vi "Periodic Tasks.vi"(8 "error in":errorcluster) -> ()   [LabVIEW 2015]
doc: "This VI runs in parallel to other tasks. It can contain as many user-defined periodic loops as you need. These can carry out PID or other sorts of timed response."
uses:
  PID Constants.ctl
  Pneumatic State Machine.ctl
  DriveStates.ctl
  DriveTypes.ctl
  Auto Control.ctl
  <vilib>/Rock Robotics/WPI/DriverStation/WPI_DriverStationAllianceInfo.ctl
  <vilib>/Rock Robotics/WPI/DriverStation/WPI_DriverStationPositionInfo.ctl
  IMUType.ctl
  <vilib>/Platform/TimedLoop/XDataNode/timing_clust.ctl
  <vilib>/Platform/TimedLoop/XDataNode/nitl_modes.ctl
  <vilib>/Platform/TimedLoop/XDataNode/wakeup.ctl
  <vilib>/Rock Robotics/WPI/Solenoid/WPI_SolenoidValue.ctl
  Pneumatic Commands.ctl
  <vilib>/Rock Robotics/WPI/DriverStation/WPI_DriverStationRobotMode2.ctl
  <vilib>/Rock Robotics/WPI/Utilities/WPI_GetSetVariantRefNum.vi
  <vilib>/Rock Robotics/WPI/Solenoid/WPI_SolenoidSetEnum.vi
  <vilib>/Rock Robotics/Network Tables/NT Write Boolean.vi
  <vilib>/Rock Robotics/Network Tables/NT Write Number.vi
  <vilib>/platform/TimedLoop/XDataNode/XDataNode.xnode
  <vilib>/addons/control/pid/NI_PID_pid.lvlib
  <vilib>/Platform/TimedLoop/XDataNode/XDNodeRunTimeDep.lvlib
  <vilib>/addons/control/pid/pid.llb/PID Output Rate Limiter (DBL).vi
  <vilib>/Rock Robotics/Network Tables/NT Read String.vi
panel:
  out "IMU Type":T1
  out "Analog Pitch Gyro 2":dbl(graph)=-229.6875
  in  "Alt imu":bool
  in  "PImu fail":bool
  out "Climb State":T2=enum."Up and Float"
  in  "Reload QCP":bool
  out "Position":T3
  out "Alliance":T4
  out "Distance Remaining 2":dbl
  out "Motor Current":dbl(graph)=12.625
  in  "Tab Control":T5(tab)=enum."Drive"
  out "Waveform Chart":cluster{"Double":dbl, "Double":dbl}(graph)
  in  "cluster 2":T6={"Command"=enum."Stop", "Distance"=70.0, "Angle"=75.0, "Power"=0.6}
  in  "Send Command 2":bool
  out "Auto Command":T7
  in  "Tollerances":T8={"Evaluation Period"=0.5, "Dead Zone"=1.0, "Throttle Scale"=0.7}
  in  "Drive Mode":u32
  in  "real mode":bool=TRUE
  out "Distance Remaining":dbl=100.0
  out "Delta Angle Remaining 2":dbl=0.3125
  out "Distance":T9(graph)
  out "Angle":cluster{"Angle Setpoint":dbl, "Yaw":dbl}(graph)={"Angle Setpoint"=87.11416811253483, "Yaw"=3.4375}
  in  "Negates":T10={"negate turn"=TRUE, "negate throttle"=FALSE}
  in  "Throttle Scale":dbl(knob)=0.6332538458134985 scale=0.0..1.0
  in  "Distance Delta":dbl=10.0
  in  "Angle Delta":dbl(knob)=83.67666811253483 scale=-100.0..100.0
  in  "output rate (EGU/min)":dbl(knob)=125.7747299198201 scale=0.0..200.0
  in  "Angle Wrap":bool
  in  "Eval Period (sec)":dbl(knob)=0.503724380465646 scale=0.0..1.0
  in  "tol":dbl=0.5 format="%#_13g"
  out "Shoot":bool
  in  "Period":i64=20
  out "Late?":bool
  out "Delta Angle Remaining":dbl=83.67666811253483
  in  "output range":cluster{"output high":dbl, "output low":dbl}={"output high"=1.0, "output low"=-1.0}
  out "Delta Angle Remaining 3":dbl
  out "Drive Mode 2":T11
  in  "PID Constants":T12={"Drive Distance PID"={"proportional gain (Kc)"=0.2, "integral time (Ti, min)"=0.0, "derivative time (Td, min)"=0.001}, "Drive Straight PID"={"proportional gain (Kc)"=0.035, "integral time (Ti, min)"=0.0, "derivative time (Td, min)"=0.0008}, "TurnPID"={"proportional gain (Kc)"=0.07, "integral time (Ti, min)"=0.005, "derivative time (Td, min)"=0.0008}, "Hold Position PID"={"proportional gain (Kc)"=0.2, "integral time (Ti, min)"=0.02, "derivative time (Td, min)"=0.001}} {"Hold Position PID"."derivative time (Td, min)" format="%.10f"; "Hold Position PID"."integral time (Ti, min)" format="%.8f"; "Hold Position PID"."proportional gain (Kc)" format="%.3f"; "TurnPID"."derivative time (Td, min)" format="%.6f"; "TurnPID"."integral time (Ti, min)" format="%.10f"; "TurnPID"."proportional gain (Kc)" format="%.6f"; "Drive Straight PID"."derivative time (Td, min)" format="%.6f"; "Drive Straight PID"."integral time (Ti, min)" format="%.10f"; "Drive Straight PID"."proportional gain (Kc)" format="%.6f"; "Drive Distance PID"."derivative time (Td, min)" format="%.10f"; "Drive Distance PID"."integral time (Ti, min)" format="%.8f"; "Drive Distance PID"."proportional gain (Kc)" format="%.3f"}
  out "M":T13={"Boolean"=FALSE, "Boolean 2"=FALSE, "Boolean 3"=FALSE, "Boolean 4"=TRUE}
  out "A":T13={"Boolean"=FALSE, "Boolean 2"=FALSE, "Boolean 3"=TRUE, "Boolean 4"=FALSE}
  out "G":T13={"Boolean"=TRUE, "Boolean 2"=FALSE, "Boolean 3"=FALSE, "Boolean 4"=FALSE}
  out "S":T13={"Boolean"=FALSE, "Boolean 2"=FALSE, "Boolean 3"=FALSE, "Boolean 4"=TRUE}
  out "Analog Yaw Gyro":dbl(graph)=-229.6875
  in  "Read Enable":T14={"Cal Status"=TRUE, "Orientation"=TRUE, "Gyro"=FALSE, "Accelerometer"=FALSE, "Quanterion"=FALSE, "Accel Mode"=enum."Linear", "Magnetometer"=FALSE}
  out "Yaw":dbl(graph)=37.4375
  out "Pitch":dbl(graph)=1.75
  out "Roll":dbl(graph)=0.5
  out "X Acc":dbl
  out "Y Acc":dbl
  out "Z Acc":dbl
  out "Anomaly":bool
  in  "Earth Field (uT)":cluster{"Earth":dbl, "Tolerance":dbl}={"Earth"=51.0, "Tolerance"=5.0}
  out "Mag Vector":dbl
  out "IMUStatus":bool
  out "Late? 2":bool
  in  "Sensor Period":i64=20
  out "pitch":dbl=1.75
  in  "Max Val":dbl(knob)=1.0 scale=0.5..1.0
  in  "Offset 2":dbl(knob)=0.6008653928286186 scale=0.0..1.0
  in  "Dead Zone 2":dbl(knob)=0.09984207295572244 scale=0.0..1.0
  in  "Offset":dbl(knob)=0.267936230826254 scale=0.0..1.0
  in  "Dead Zone":dbl(knob)=0.10126960022109426 scale=0.0..1.0
  out "Left Encoder Distance":dbl=4402.950615
  out "Right Encoder Distance":dbl
  in  "Reset Encoders":bool
  out "Intake Chart":dbl(graph)=3.0
  out "Intake State":T2=enum."Up and Float"
  out "Tusk State":T2=enum."Up and Float"
  in  "a parameter too":dbl=0.5 format="%#_13g"
  in  "dist away":dbl=20.0 format="%#_13g"
  out "pitch 2":dbl=1.75
  out "Mag Vector 2":dbl
  out "Anomaly 2":bool
  in  "Earth Field (uT) 2":cluster{"Earth":dbl, "Tolerance":dbl}={"Earth"=51.0, "Tolerance"=5.0}
  out "Z Acc 2":dbl
  out "Y Acc 2":dbl
  out "X Acc 2":dbl
  out "M 2":T13={"Boolean"=FALSE, "Boolean 2"=FALSE, "Boolean 3"=FALSE, "Boolean 4"=TRUE}
  out "A 2":T13={"Boolean"=FALSE, "Boolean 2"=FALSE, "Boolean 3"=TRUE, "Boolean 4"=FALSE}
  out "G 2":T13={"Boolean"=TRUE, "Boolean 2"=FALSE, "Boolean 3"=FALSE, "Boolean 4"=FALSE}
  out "S 2":T13={"Boolean"=FALSE, "Boolean 2"=FALSE, "Boolean 3"=FALSE, "Boolean 4"=TRUE}
  in  "Read Enable 2":T14={"Cal Status"=TRUE, "Orientation"=TRUE, "Gyro"=FALSE, "Accelerometer"=FALSE, "Quanterion"=FALSE, "Accel Mode"=enum."Linear", "Magnetometer"=FALSE}
  # "Bazemore\nStraight Gains\nP=0.035\nI=0.00\nD=0.0008"
  # "Cass\nHold Position\nGains\nP=0.2\nI=0.02\nD=0.001"
  # "Bazemore\nTurn Gains\nP=0.07\nI=0.005\nD=0.0008"
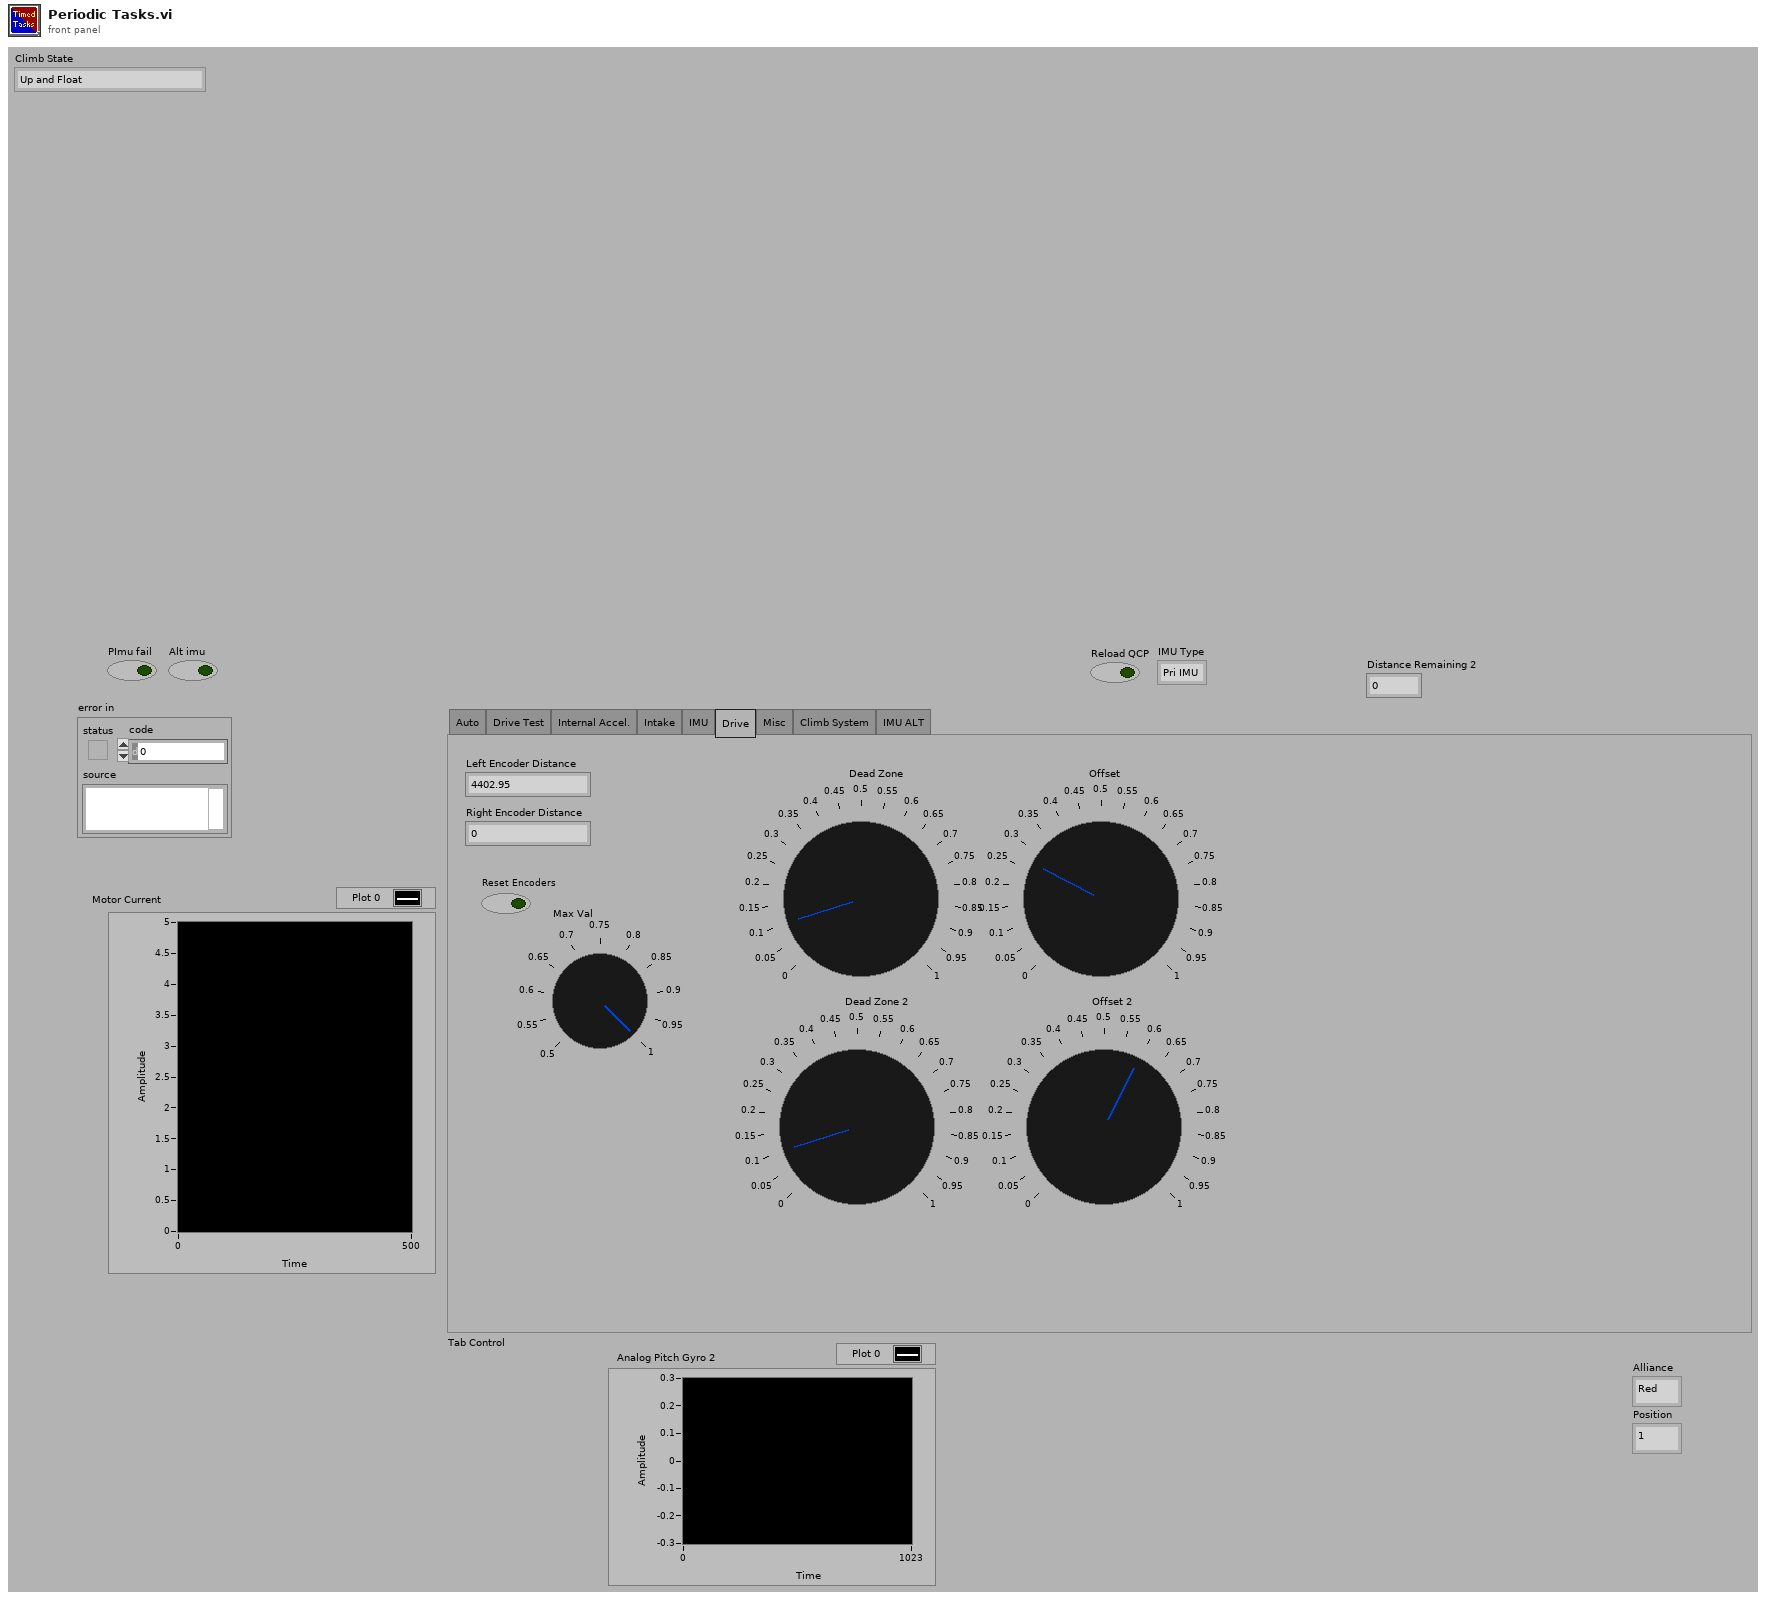
[diagram p1: front panel]
types:
  T1 = typedef "IMUType.ctl" = enum16{"Pri IMU", "Alt IMU", "Analog GYRO"}
  T2 = typedef "Pneumatic State Machine.ctl" = enum16{"Up and Pressure", "Down and Pressue", "Up and Float", "Down and Float"}
  T3 = typedef "WPI_DriverStationPositionInfo.ctl" = enum16{"1", "2", "3"}
  T4 = typedef "WPI_DriverStationAllianceInfo.ctl" = enum16{"Red", "Blue", "Invalid"}
  T5 = enum32{"Auto", "Drive Test", "Internal Accel.", "Intake", "IMU", "Drive", "Misc", "Climb System", "IMU ALT"}
  T6 = typedef "Auto Control.ctl" = cluster{"Command":T7, "Distance":dbl, "Angle":dbl, "Power":dbl}
  T7 = typedef "DriveStates.ctl" = enum16{"Wait for Notification", "Drive for Distance", "Drive Continuous", "Drive Absolute Heading", "Drive Relative Heading", "Turn Continuous", "Turn Degree", "Stop", "Follow Camera", "Hold Position"}
  T8 = cluster{"Evaluation Period":dbl, "Dead Zone":dbl, "Throttle Scale":dbl}
  T9 = cluster{"Distance Setpoint":dbl, "Desired Distance":dbl}
  T10 = cluster{"negate turn":bool, "negate throttle":bool}
  T11 = typedef "DriveTypes.ctl" = enum16{"Auto Turn", "Auto Straight", "Auto Vision Align"}
  T12 = typedef "PID Constants.ctl" = cluster{"Drive Distance PID":cluster{"proportional gain (Kc)":dbl, "integral time (Ti, min)":dbl, "derivative time (Td, min)":dbl}, "Drive Straight PID":cluster{"proportional gain (Kc)":dbl, "integral time (Ti, min)":dbl, "derivative time (Td, min)":dbl}, "TurnPID":cluster{"proportional gain (Kc)":dbl, "integral time (Ti, min)":dbl, "derivative time (Td, min)":dbl}, "Hold Position PID":cluster{"proportional gain (Kc)":dbl, "integral time (Ti, min)":dbl, "derivative time (Td, min)":dbl}}
  T13 = cluster{"Boolean":bool, "Boolean 2":bool, "Boolean 3":bool, "Boolean 4":bool}
  T14 = cluster{"Cal Status":bool, "Orientation":bool, "Gyro":bool, "Accelerometer":bool, "Quanterion":bool, "Accel Mode":enum8{"Raw Data", "Linear", "Gravity"}, "Magnetometer":bool}
  T15 = cluster{"Yaw Wind":dbl, "Roll Wind":dbl, "Pitch Wind":dbl}
  T16 = typedef "WPI_DriverStationRobotMode2.ctl" = enum16{"Autonomous Disabled", "Autonomous Enabled", "Teleop Disabled", "Teleop Enabled", "Disconnected", "Finish", "Test Disabled", "Test Enabled", "Emergency Stopped"}
  T17 = typedef "Pneumatic Commands.ctl" = enum16{"Go Up", "Go Down", "Nothing"}
  T18 = typedef "WPI_SolenoidValue.ctl" = enum16{"Off", "On", "Forward", "Reverse"}
  T19 = cluster{"tdms":refnum<k34>, "Channel IDs":string[], "TDMS Name":string, "Burst Size":i32, "Que":refnum<k33>, "Default Array":dbl[], "occurrence":refnum<k4>}
  T20 = typedef "XDNodeRunTimeDep.lvlib/timing_clust.ctl" = cluster{"Expected End [f-1]":u64, "Actual End [f-1]":u64, "Finished Late? [f-1]":bool, "Expected End [i-1]":u64, "Actual End [i-1]":u64, "Finished Late? [i-1]":bool, "Expected Start [i]":u64, "Actual Start [i]":u64, "Expected Start [f]":u64, "Actual Start [f]":u64, "Source Name":string, "Structure Name":string, "Period":i64, "Deadline":i64, "Offset":i64, "Start":i64, "Priority":i32, "Timeout":i32, "Mode":T21, "Wakeup Reason":T22, "Error":errorcluster, "Source Type":string, "Secondary Source Type":string, "Global End Time":u64, "Global Start Time":u64, "Frame Duration":u64, "Iteration Duration":u64, "Assigned CPU":i32, "I/O Scan Engine Mode":u32}
  T21 = typedef "XDNodeRunTimeDep.lvlib/nitl_modes.ctl" = enum32{"No Change", "Process missed periods, maintain original phase", "Discard missed periods, maintain original phase", "Process missed periods, ignore original phase", "Discard missed periods, ignore original phase"}
  T22 = typedef "XDNodeRunTimeDep.lvlib/wakeup.ctl" = enum32{"Normal", "Aborted", "Asynchronous wakeup", "Timing source error", "Timed loop error", "Timeout"}
  T23 = enum16{"Low Bar", "Rough Terrain", "Moat", "Rock Wall", "Cheval de Frise", "Portcullis", "Sally Port", "Drawbridge", "Ramparts"}
  T24 = typedef "WPI_JoystickDevRef.ctl" = cluster{"Device":T25}
  T25 = typedef "WPI_JoystickDeviceEnum.ctl" = enum16{"USB 0", "USB 1", "USB 2", "USB 3", "USB 4", "USB 5"}
  T26 = typedef "WPI_RobotDriveDevRef.ctl" = cluster{"DevStatus":errorcluster, "Motors[]":T27[], "Square Inputs":bool, "Max Output":dbl}
  T27 = typedef "WPI_MotorControlDeviceRef.ctl" = cluster{"DeviceStatus":errorcluster, "Type":T28, "PWM":cluster{"PWM Channel":T29, "DeadBand":T30}, "CAN":cluster{"Device Number":u8, "Control Mode":T31, "Semaphore":T32, "Max Vout":dbl, "TalonSRX Control Mode":T33}, "Invert":bool}
  T28 = typedef "WPI_MotorControlType.ctl" = enum16{"PWM", "CAN", "CANTalonSRX"}
  T29 = typedef "FPGA_DIOPWMChannel.ctl" = enum8{"PWM 0", "PWM 1", "PWM 2", "PWM 3", "PWM 4", "PWM 5", "PWM 6", "PWM 7", "PWM 8", "PWM 9", "PWM MXP 0", "PWM MXP 1", "PWM MXP 2", "PWM MXP 3", "PWM MXP 4", "PWM MXP 5", "PWM MXP 6", "PWM MXP 7", "PWM MXP 8", "PWM MXP 9", "Invalid"}
  T30 = typedef "WPI_PWMDeadband.ctl" = cluster{"Name":string, "maxPositivePwm":i32, "minPositivePwm":i32, "centerPwm":i32, "maxNegativePwm":i32, "minNegativePwm":i32, "angularRange":u16}
  T31 = typedef "WPI_CANJaguar_ControlMode.ctl" = enum8{"Percent VBus", "Current", "Speed", "Position", "Voltage"}
  T32 = typedef "Semaphore RefNum" = refnum<k1>
  T33 = typedef "WPI_CANTalonSRX_APIControlMode.ctl" = enum8{"Percent VBus", "Speed", "Position", "Slave", "Unchanged / Invalid", "Voltage Compensation", "Current", "Motion Profile"}
  T34 = cluster{"Delta":dbl, "Throttle Scale":dbl, "Current Angle":dbl, "Current Distance":dbl}
  T35 = cluster{"Buttons[0]":bool, "Buttons[1]":bool, "Buttons[2]":bool, "Buttons[3]":bool, "Buttons[4]":bool, "Buttons[5]":bool, "Buttons[6]":bool, "Buttons[7]":bool, "Buttons[8]":bool}
  T36 = cluster{"Axes[0]":dbl, "Axes[1]":dbl, "Axes[2]":dbl, "Axes[3]":dbl, "Axes[4]":dbl, "Axes[5]":dbl, "Axes[6]":dbl, "Axes[7]":dbl, "Axes[8]":dbl}
  T37 = cluster{"proportional gain (Kc)":dbl, "integral time (Ti, min)":dbl, "derivative time (Td, min)":dbl}
  T38 = cluster{"Drive Distance PID":cluster{"proportional gain (Kc)":dbl, "integral time (Ti, min)":dbl, "derivative time (Td, min)":dbl}, "Drive Straight PID":cluster{"proportional gain (Kc)":dbl, "integral time (Ti, min)":dbl, "derivative time (Td, min)":dbl}}
  T39 = cluster{"Angle Setpoint":dbl, "Distance Setpoint":dbl}
  T40 = cluster{"Distance Setpoint":dbl, "Current Distance":dbl}
  T41 = typedef "WPI_I2CDevRef.ctl" = cluster{"DevStatus":errorcluster, "Device Address":u8, "Handle":i32, "I2C Bus":T42}
  T42 = typedef "i2c_bus.ctl" = enum16{"I2C On-Board", "I2C MXP", "Invalid"}
  T43 = typedef "WPI_GyroDevRef.ctl" = cluster{"DevStatus":errorcluster, "Analog Channel":T44, "Offset":dbl, "Gain (VoltsPerDegree/Second)":dbl, "Gyro Type":enum16{"Analog", "XRS450"}, "Handle":i32, "SPI Bus":T45, "Device Found":bool, "Sample Rate":dbl, "Calibrate On Open":bool}
  T44 = typedef "FPGA_AIChannel.ctl" = enum8{"AI 0", "AI 1", "AI 2", "AI 3", "AI MXP 0", "AI MXP 1", "AI MXP 2", "AI MXP 3", "Invalid"}
  T45 = typedef "spi_bus.ctl" = enum16{"SPI On-Board, CS0", "SPI On-Board, CS1", "SPI On-Board, CS2", "SPI On-Board, CS3", "SPI MXP", "Invalid"}
  T46 = typedef "WPI_ServoDeviceRef.ctl" = cluster{"DeviceStatus":errorcluster, "PWM Channel":T29, "DeadBand":T30}
  T47 = typedef "WPI_SolenoidDevRef.ctl" = cluster{"DevStatus":errorcluster, "Pneumatics Control Module":u8, "Forward Solenoid Channel":T48, "Reverse Solenoid Channel":T48}
  T48 = typedef "WPI_SolenoidChannel.ctl" = enum8{"Solenoid 0", "Solenoid 1", "Solenoid 2", "Solenoid 3", "Solenoid 4", "Solenoid 5", "Solenoid 6", "Solenoid 7", "Invalid"}
  T49 = cluster{"Mag":cluster{"[0]":bool, "[1]":bool, "[2]":bool, "[3]":bool}, "Acc":cluster{"[0]":bool, "[1]":bool, "[2]":bool, "[3]":bool}, "Gyro":cluster{"[0]":bool, "[1]":bool, "[2]":bool, "[3]":bool}, "Sys":cluster{"[0]":bool, "[1]":bool, "[2]":bool, "[3]":bool}, "Status":bool}
  T50 = cluster{"Yaw":dbl, "Roll":dbl, "Pitch":dbl, "Yaw Wind":dbl, "Roll Wind":dbl, "Pitch Wind":dbl}
  T51 = cluster{"X Mag":dbl, "Y Mag":dbl, "Z Mag":dbl, "Anomaly":bool}
  T52 = cluster{"[0]":bool, "[1]":bool, "[2]":bool, "[3]":bool}
  T53 = typedef "WPI_EncoderDevRef.ctl" = cluster{"DevStatus":errorcluster, "EncoderIndex":T54, "CounterIndex":T55, "DistancePerCount":dbl, "Decoding Type":T56}
  T54 = typedef "FPGA_EncoderIdx.ctl" = enum8{"Enc 0", "Enc 1", "Enc 2", "Enc 3", "Enc 4", "Enc 5", "Enc 6", "Enc 7", "Invalid"}
  T55 = typedef "FPGA_CounterCtrSystemIndex.ctl" = enum8{"Ctr 0", "Ctr 1", "Ctr 2", "Ctr 3", "Ctr 4", "Ctr 5", "Ctr 6", "Ctr 7", "Invalid"}
  T56 = typedef "WPI_EncoderType.ctl" = enum16{"1x", "2x", "4x"}
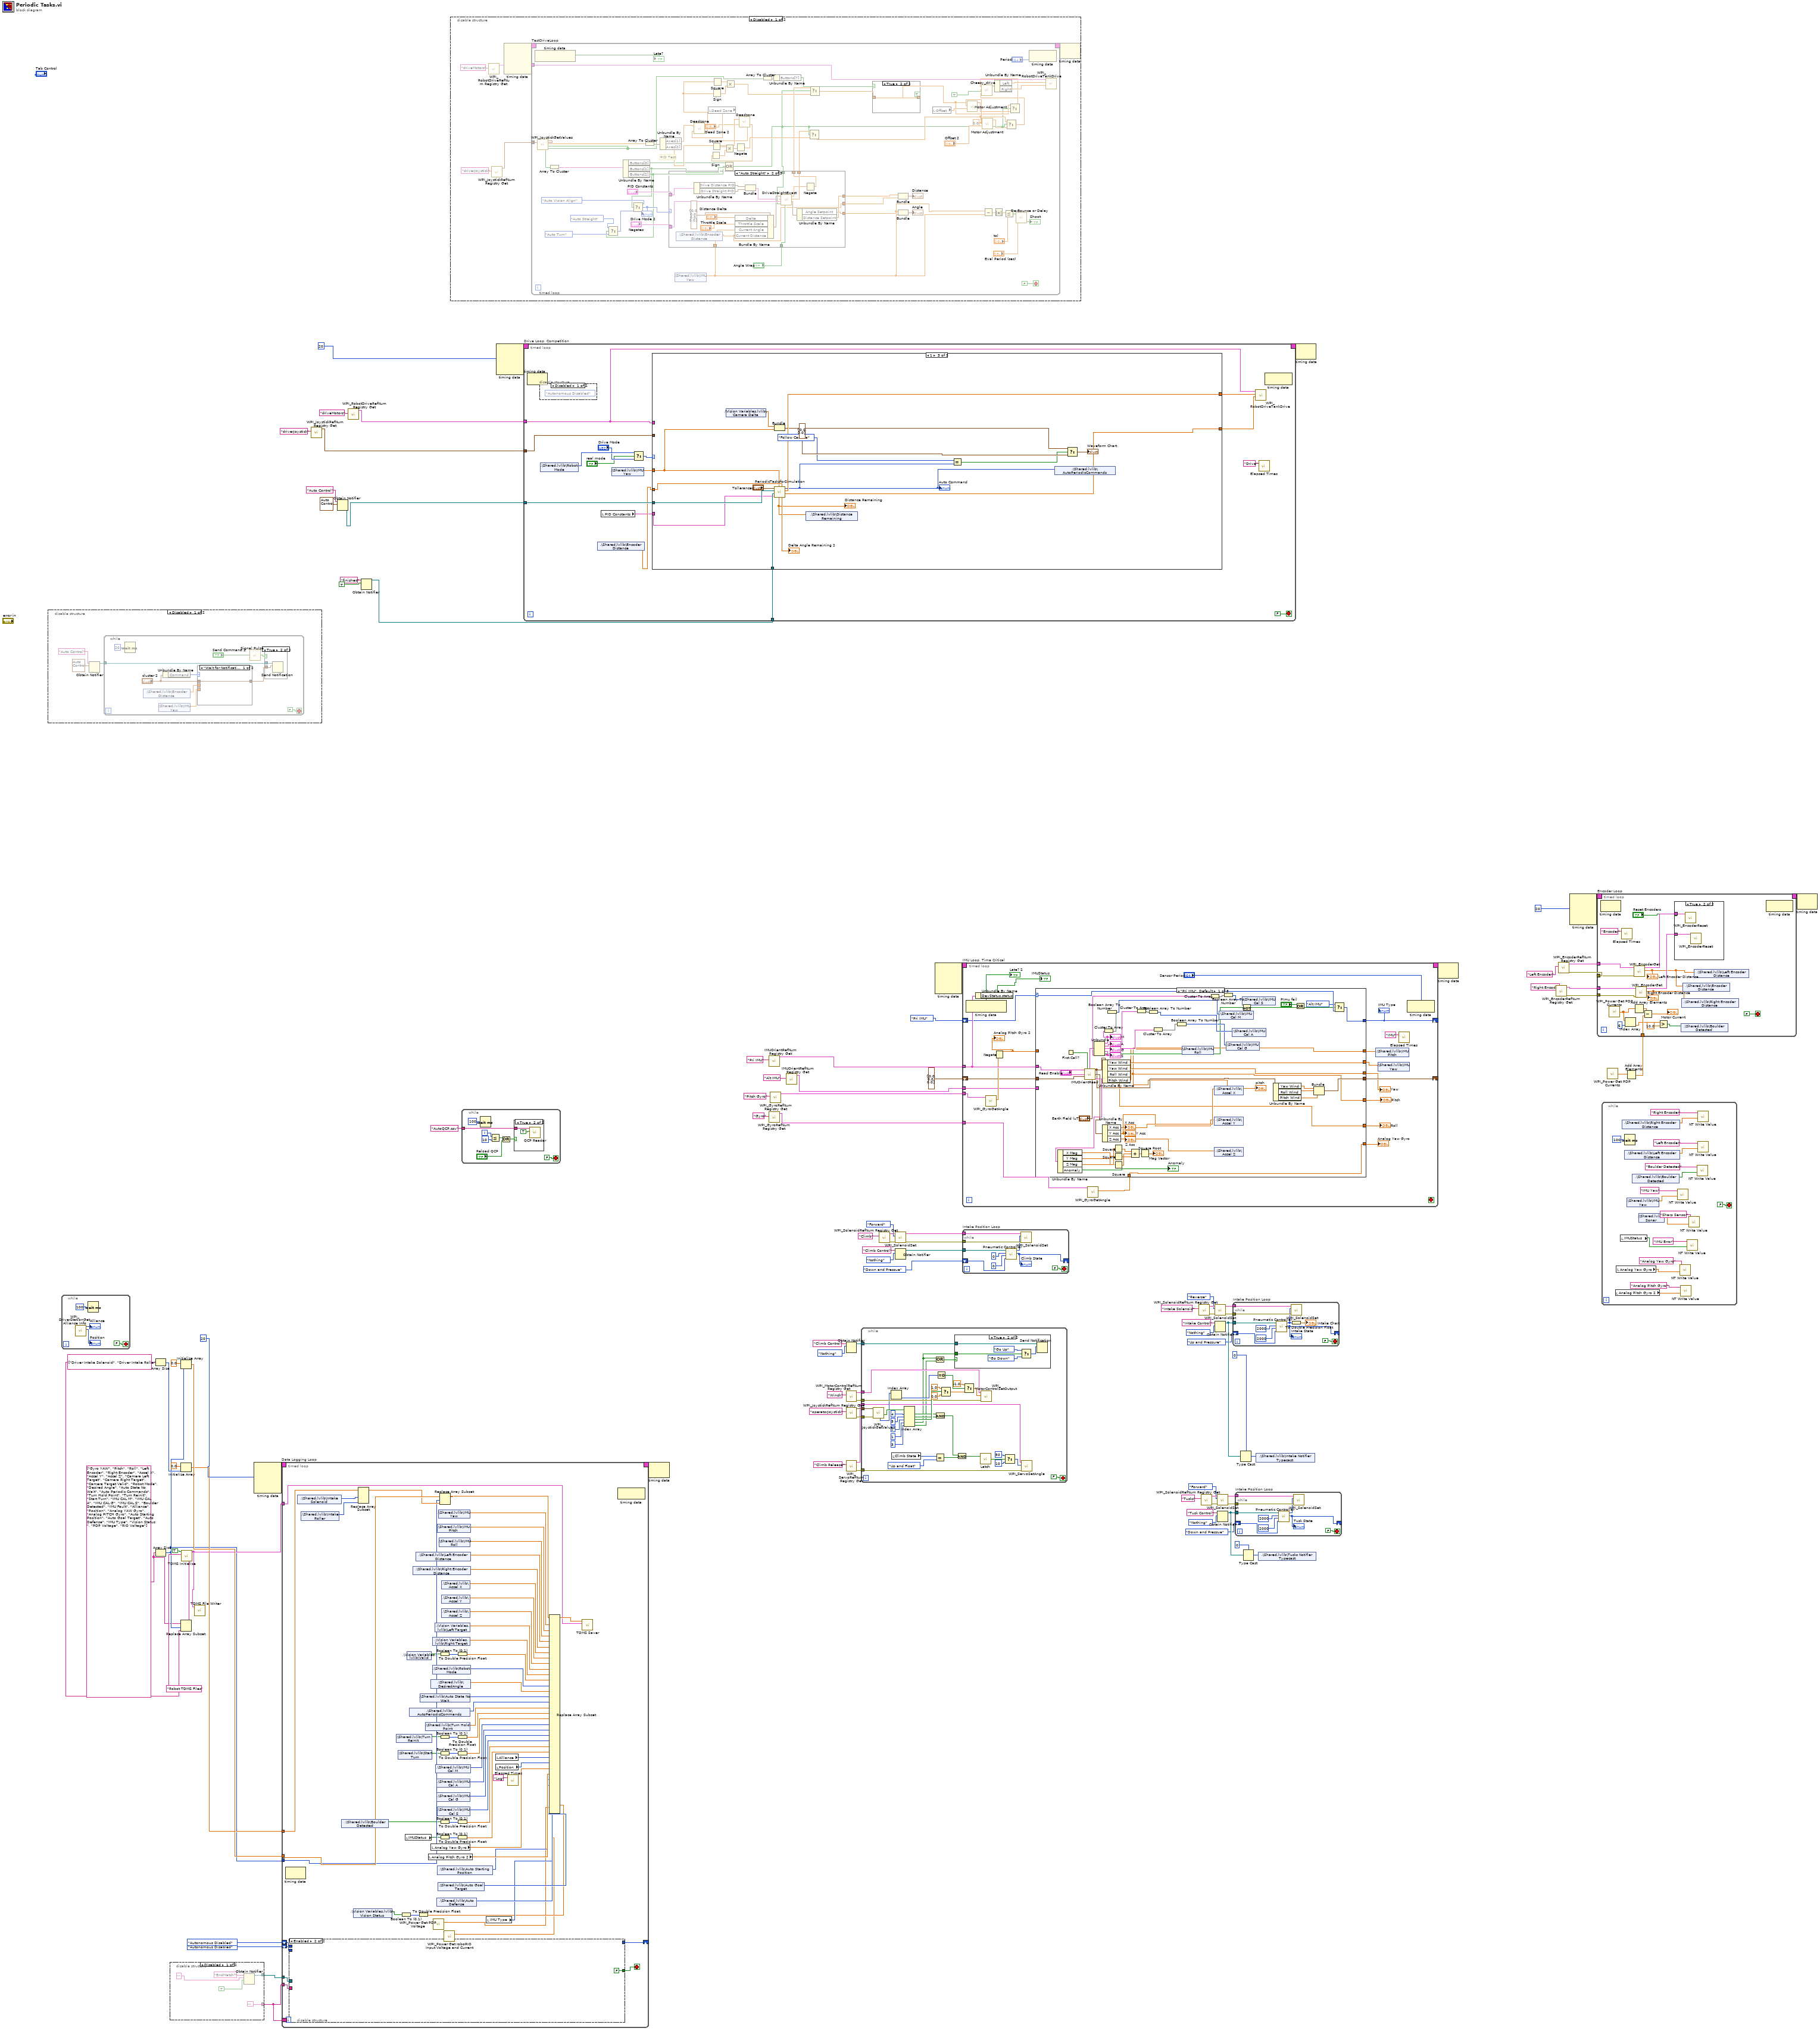
[diagram p0: block diagram]
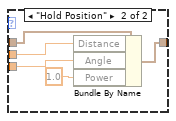
[diagram p4: hidden frame]
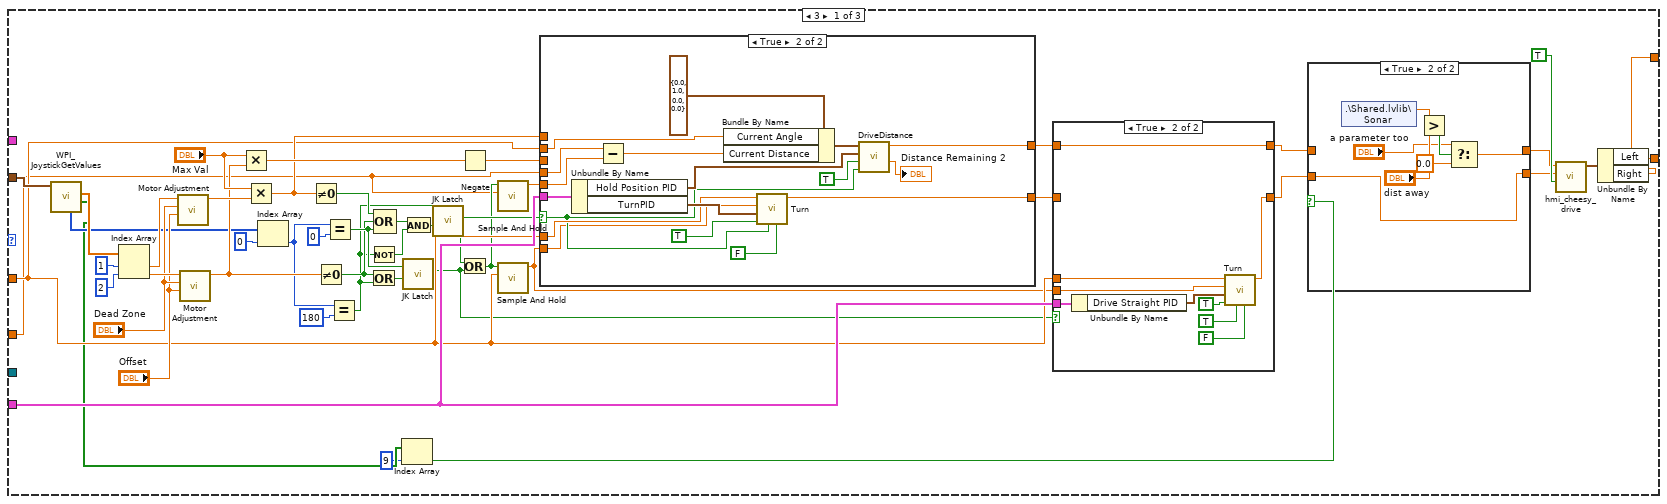
[diagram p9: hidden frame]
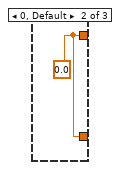
[diagram p13: hidden frame]
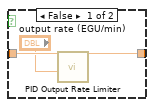
[diagram p14: hidden frame]
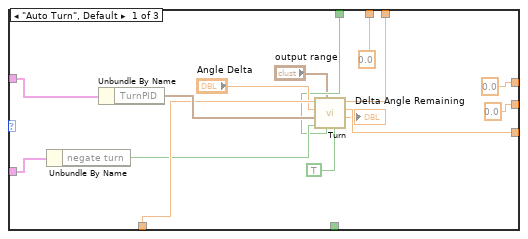
[diagram p15: hidden frame]
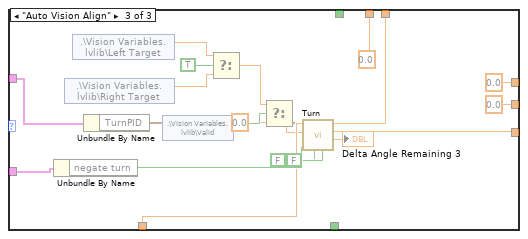
[diagram p16: hidden frame]
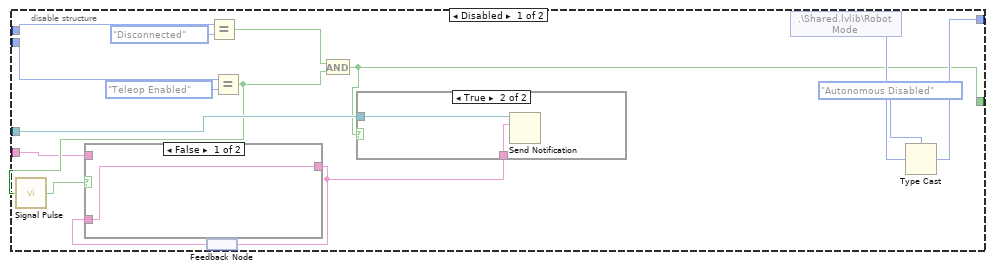
[diagram p19: hidden frame]
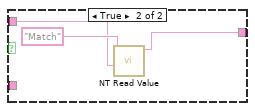
[diagram p20: hidden frame]
diagram:
  w1 = string[] ["Driver Intake Solenoid", "Driver Intake Roller"] ("Channel IDs")
  w3 = string[] ["Gyro YAW", "Pitch", "Roll", "Left Encoder", "Right Encoder", "Accel X", "Accel Y", "Accel Z", "Camera Left Target", "Camera Right Target", "Camera Target Valid", "Robot Mode", "Desired Angle", "Auto State No Wait", "Auto Periodic Commands", "Turn Hold Point", "Turn Reinit", "Start Turn", "IMU CAL M", "IMU CAL A", "IMU CAL G", "IMU CAL S", "Boulder Detected", "IMU Fault", "Alliance", "Position", "Analog YAW Gyro", "Analog PITCH Gyro", "Auto Starting Position", "Auto Goal Target", "Auto Defense", "IMU Type", "Vision Status ", "PDP Voltage", "RIO Voltage"] ("Channel IDs")
  n1 = disable-structure shown="Disabled" {
    frame Disabled {
      n2 = Obtain Notifier(name (unnamed)="Auto Control", notification data type=T6 {"Command"=enum."Drive for Distance", "Distance"=0.0, "Angle"=0.0, "Power"=0.0} ("cluster")) -> (notifier out=w103:refnum<notifier>)  [unwired: 2 in, 2 out]
      n3 = while {
        tunnel: w103 -> [w113]
        stop <- FALSE stop-if-true
        n4 = Wait (ms)(milliseconds to wait=u32 20) -> ()  [unwired: 1 out]
        n5 = shared-variable ".\\Shared.lvlib\\Encoder Distance"() -> (w107:dbl)  [unwired: 1 in, 1 out]
        n6 = shared-variable ".\\Shared.lvlib\\IMU Yaw"() -> (w106:dbl)  [unwired: 1 in, 1 out]
        n7 = Unbundle By Name("cluster 2") -> ("Command"=w110:T7)
        n8 = case shown="\"Wait for Notification\", Default" w110 {
          tunnel: "cluster 2" -> [w116 w121]
          tunnel: [w116 w120] -> w108
          tunnel: w107 -> [_ w119]
          tunnel: w106 -> [_ w118]
          frame "Wait for Notification", Default {
          }
          frame "Hold Position" {
            n9 = Bundle By Name(cluster=w121, "Distance"=w119, "Angle"=w118, "Power"=1.0) -> (w120:T6)
          }
        }
        n10 = call <userlib>:"Signal Pulse.vi"("Input"="Send Command 2") -> ("Output"=w114:bool)
        n11 = case shown="True" w114 {
          tunnel: w113 -> [_ w123]
          tunnel: w108 -> [_ w122]
          frame False {
          }
          frame True {
            n12 = Send Notification(notification=w122, notifier=w123) -> ()  [unwired: 1 in, 2 out]
          }
        }
      }
    }
    frame Enabled {
    }
  }
  n13 = while {
    stop <- FALSE stop-if-true
    n14 = call <vilib>:"WPI_DriverStationGet Alliance Info.vi"() -> ("Position"=→"Position":T3, "Alliance"=→"Alliance":T4)  [unwired: 10 in]
    n15 = Wait (ms)(milliseconds to wait=u32 100) -> ()  [unwired: 1 out]
  }
  n16 = Array Size(array=w1) -> (size(s)=w74:i32)
  n17 = Array Size(array=w3) -> (size(s)=w4:i32)
  n18 = disable-structure shown="Disabled" {
    disable-tunnel: [w130 _] -> w9
    disable-tunnel: ["" _] -> w8
    frame Disabled {
      n19 = Obtain Notifier(name (unnamed)="EndMatch?", notification data type="", create if not found? (T)=TRUE) -> (notifier out=w130:refnum<notifier>)  [unwired: 1 in, 2 out]
    }
    frame Enabled {
    }
  }
  n20 = Initialize Array(0.0, w4) -> (w89:dbl[])
  n21 = Initialize Array(0.0, w74) -> (w73:dbl[])
  n22 = Replace Array Subset(array=w3, new element=w1, index=w4) -> (w2:string[])
  n23 = call <userlib>:"TDMS Initialize.vi"("Channel IDs"=w2, "TDMS Name"="Robot TDMS Files", "Log to USB?"=TRUE) -> ("TDMS Cluster"=w5:T19)  [unwired: 8 in]
  n24 = call <userlib>:"TDMS File Writer.vi"("TDMS Cluster"=w5) -> ()  [unwired: 11 in]
  n25 = node-c288(i64 20 ("Period")) -> (w94:T20)  [unwired: 3 in]
  n26 = timed-loop "Data Logging Loop" {
    timing: w94 -> [_]
    timing-out: [_] -> w93
    tunnel: w5 -> [w170]
    tunnel: w89 -> [w186]
    tunnel: w73 -> [w184]
    tunnel: w4 -> [w182]
    shift-right: [w146] -> _
    shift-left: WPI_DriverStationRobotMode2."Autonomous Disabled" ("Robot Mode") -> [w148]
    shift-left: WPI_DriverStationRobotMode2."Autonomous Disabled" ("Robot Mode") -> [w147]
    tunnel: w9 -> [w145]
    border: w8 -> [_]
    tunnel: w8 -> [w143]
    stop <- w144 stop-if-true
    n27 = node-c288() -> ()  [unwired: 1 in, 1 out]
    n28 = disable-structure shown="Enabled" {
      disable-tunnel: w148 -> [w210 _]
      disable-tunnel: w147 -> [w209 _]
      disable-tunnel: [w207 _] -> w146
      disable-tunnel: w145 -> [w202 _]
      disable-tunnel: [w201 FALSE] -> w144
      disable-tunnel: w143 -> [w197 _]
      frame Disabled {
        n29 = feedback #1() -> (w198:string)
        n30 = Equal?(x=w210, y=WPI_DriverStationRobotMode2."Disconnected") -> (x = y?=w203:bool)
        n31 = Equal?(x=w209, y=WPI_DriverStationRobotMode2."Teleop Enabled") -> (x = y?=w200:bool)
        n32 = call <userlib>:"Signal Pulse.vi"("Input"=w200) -> ("Output"=w199:bool)
        n33 = case shown="False" w199 {
          tunnel: [w211 w213] -> w196
          tunnel: w197 -> [_ w212]
          tunnel: w198 -> [w211 _]
          frame False {
          }
          frame True {
            n34 = call-poly <vilib>:"NT Read Value.vi"("Default Value"=w212, "Name"="Match") -> ("String"=w213:string)  [unwired: 8 in, 1 out]
          }
        }
        n35 = feedback-in #1(w196) -> ()
        n36 = And(x=w203, y=w200) -> (x .and. y?=w201:bool)
        n37 = case shown="True" w201 {
          tunnel: w202 -> [_ w216]
          tunnel: w196 -> [_ w215]
          frame False {
          }
          frame True {
            n38 = Send Notification(notification=w215, notifier=w216) -> ()  [unwired: 1 in, 2 out]
          }
        }
        n39 = shared-variable ".\\Shared.lvlib\\Robot Mode"() -> (w208:u32)  [unwired: 1 in, 1 out]
        n40 = Type Cast(type=WPI_DriverStationRobotMode2."Autonomous Disabled" ("Robot Mode"), x=w208) -> (*(type *) &x=w207:T16)
      }
      frame Enabled {
      }
    }
    n41 = shared-variable ".\\Shared.lvlib\\Intake Solenoid"() -> (w181:u32)  [unwired: 1 in, 1 out]
    n42 = shared-variable ".\\Shared.lvlib\\Intake Roller"() -> (w180:u32)  [unwired: 1 in, 1 out]
    n43 = shared-variable ".\\Shared.lvlib\\Boulder Detected"() -> (w158:bool)  [unwired: 1 in, 1 out]
    n44 = shared-variable ".\\Vision Variables.lvlib\\Vision Status"() -> (w136:bool)  [unwired: 1 in, 1 out]
    n45 = Replace Array Subset(array=w184, new element #1=w181, new element #2=w180) -> (w183:dbl[])  [unwired: 2 in]
    n46 = shared-variable ".\\Shared.lvlib\\Turn Reinit"() -> (w167:bool)  [unwired: 1 in, 1 out]
    n47 = shared-variable ".\\Shared.lvlib\\Start Turn"() -> (w165:bool)  [unwired: 1 in, 1 out]
    n48 = Boolean To (0,1)(Boolean=w136) -> (0, 1=w137:i16)
    n49 = local read "IMUStatus"() -> (w151:bool)
    n50 = shared-variable ".\\Vision Variables.lvlib\\Valid"() -> (w177:bool)  [unwired: 1 in, 1 out]
    n51 = shared-variable ".\\Shared.lvlib\\AutoPeriodicCommands"() -> (w171:u16)  [unwired: 1 in, 1 out]
    n52 = shared-variable ".\\Shared.lvlib\\Right Encoder Distance"() -> (w190:dbl)  [unwired: 1 in, 1 out]
    n53 = shared-variable ".\\Shared.lvlib\\Left Encoder Distance"() -> (w191:dbl)  [unwired: 1 in, 1 out]
    n54 = To Double Precision Float(number=w137) -> (double precision float=w135:dbl)
    n55 = shared-variable ".\\Shared.lvlib\\Auto State No Wait"() -> (w172:u32)  [unwired: 1 in, 1 out]
    n56 = shared-variable ".\\Shared.lvlib\\Turn Hold Point"() -> (w169:dbl)  [unwired: 1 in, 1 out]
    n57 = local read "Analog Pitch Gyro 2"() -> (w142:dbl)
    n58 = shared-variable ".\\Shared.lvlib\\DesiredAngle"() -> (w173:dbl)  [unwired: 1 in, 1 out]
    n59 = local read "Analog Yaw Gyro"() -> (w149:dbl)
    n60 = shared-variable ".\\Vision Variables.lvlib\\Right Target"() -> (w178:dbl)  [unwired: 1 in, 1 out]
    n61 = shared-variable ".\\Shared.lvlib\\Robot Mode"() -> (w174:u32)  [unwired: 1 in, 1 out]
    n62 = call <vilib>:"WPI_Power Get PDP Voltage.vi"() -> ("voltage (V)"=w134:dbl)  [unwired: 14 in, 1 out]
    n63 = shared-variable ".\\Vision Variables.lvlib\\Left Target"() -> (w179:dbl)  [unwired: 1 in, 1 out]
    n64 = shared-variable ".\\Shared.lvlib\\IMU Cal M"() -> (w162:u32)  [unwired: 1 in, 1 out]
    n65 = shared-variable ".\\Shared.lvlib\\IMU Cal A"() -> (w161:u32)  [unwired: 1 in, 1 out]
    n66 = shared-variable ".\\Shared.lvlib\\IMU Cal G"() -> (w160:u32)  [unwired: 1 in, 1 out]
    n67 = shared-variable ".\\Shared.lvlib\\Auto Defense"() -> (w139:T23)  [unwired: 1 in, 1 out]
    n68 = shared-variable ".\\Shared.lvlib\\IMU Pitch"() -> (w193:dbl)  [unwired: 1 in, 1 out]
    n69 = shared-variable ".\\Shared.lvlib\\IMU Cal S"() -> (w159:u32)  [unwired: 1 in, 1 out]
    n70 = shared-variable ".\\Shared.lvlib\\Auto Starting Position"() -> (w141:enum16{"1", "2", "3", "4", "5"})  [unwired: 1 in, 1 out]
    n71 = shared-variable ".\\Shared.lvlib\\Auto Goal Target"() -> (w140:enum16{"Left Goal", "Right Goal", "Stop"})  [unwired: 1 in, 1 out]
    n72 = shared-variable ".\\Shared.lvlib\\IMU Yaw"() -> (w194:dbl)  [unwired: 1 in, 1 out]
    n73 = shared-variable ".\\Shared.lvlib\\IMU Roll"() -> (w192:dbl)  [unwired: 1 in, 1 out]
    n74 = Boolean To (0,1)(Boolean=w177) -> (0, 1=w176:i16)
    n75 = Boolean To (0,1)(Boolean=w167) -> (0, 1=w168:i16)
    n76 = Boolean To (0,1)(Boolean=w165) -> (0, 1=w166:i16)
    n77 = Boolean To (0,1)(Boolean=w158) -> (0, 1=w157:i16)
    n78 = Boolean To (0,1)(Boolean=w151) -> (0, 1=w152:i16)
    n79 = Replace Array Subset(array=w186, new element=w183, index=w182) -> (w185:dbl[])
    n80 = shared-variable ".\\Shared.lvlib\\Accel X"() -> (w189:dbl)  [unwired: 1 in, 1 out]
    n81 = shared-variable ".\\Shared.lvlib\\Accel Y"() -> (w188:dbl)  [unwired: 1 in, 1 out]
    n82 = shared-variable ".\\Shared.lvlib\\Accel Z"() -> (w187:dbl)  [unwired: 1 in, 1 out]
    n83 = call <vilib>:"WPI_Power Get roboRIO Input Voltage and Current.vi"() -> ("roboRIO input voltage (V)"=w133:dbl)  [unwired: 13 in, 2 out]
    n84 = To Double Precision Float(number=w176) -> (double precision float=w175:dbl)
    n85 = To Double Precision Float(number=w168) -> (double precision float=w164:dbl)
    n86 = To Double Precision Float(number=w166) -> (double precision float=w163:dbl)
    n87 = To Double Precision Float(number=w157) -> (double precision float=w156:dbl)
    n88 = To Double Precision Float(number=w152) -> (double precision float=w150:dbl)
    n89 = local read "IMU Type"() -> (w138:T1)
    n90 = local read "Alliance"() -> (w153:T4)
    n91 = local read "Position"() -> (w154:T3)
    n92 = call "Elapsed Times.vi"("Call Name"="Log") -> ()  [unwired: 2 in, 1 out]
    n93 = Replace Array Subset(array=w185, new element #1=w194, new element #2=w193, new element #3=w192, new element #4=w191, new element #5=w190, new element #6=w189, new element #7=w188, new element #8=w187, new element #9=w179, new element #10=w178, new element #11=w175, new element #12=w174, new element #13=w173, new element #14=w172, new element #15=w171, new element #16=w169, new element #17=w164, new element #18=w163, new element #19=w162, new element #20=w161, new element #21=w160, new element #22=w159, new element #23=w156, new element #24=w150, new element #25=w153, new element #26=w154, new element #27=w149, new element #28=w142, new element #29=w141, new element #30=w140, new element #31=w139, new element #32=w138, new element #33=w135, new element #34=w134, new element #35=w133) -> (w195:dbl[])  [unwired: 35 in]
    n94 = call <userlib>:"TDMS Saver.vi"("TDMS Cluster"=w170, "Data to Log"=w195) -> ()  [unwired: 10 in]
    n95 = node-c288() -> ()  [unwired: 1 in, 1 out]
  }
  n96 = call <vilib>:"WPI_JoystickRefNum Registry Get.vi"("refnum name"="driverJoystick") -> ("JoystickDevRef"=w62:T24)  [unwired: 1 in, 9 out]
  n97 = Obtain Notifier(name (unnamed)="Auto Control", notification data type=T6 {"Command"=enum."Drive for Distance", "Distance"=0.0, "Angle"=0.0, "Power"=0.0} ("cluster")) -> (notifier out=w65:refnum<notifier>)  [unwired: 2 in, 2 out]
  n98 = call <vilib>:"WPI_RobotDriveRefNum Registry Get.vi"("refnum name"="driveMotors") -> ("RobotDriveDevRef"=w67:T26)  [unwired: 9 in, 1 out]
  n99 = Obtain Notifier(name (unnamed)="finished", notification data type=TRUE) -> (notifier out=w36:refnum<notifier>)  [unwired: 2 in, 2 out]
  n100 = disable-structure shown="Disabled" {
    frame Disabled {
      n101 = call <vilib>:"WPI_RobotDriveRefNum Registry Get.vi"("refnum name"="driveMotors") -> ("RobotDriveDevRef"=w222:T26)  [unwired: 9 in, 1 out]
      n102 = call <vilib>:"WPI_JoystickRefNum Registry Get.vi"("refnum name"="driverJoystick") -> ("JoystickDevRef"=w220:T24)  [unwired: 9 in, 1 out]
      n103 = node-c288() -> (w225:T20)  [unwired: 4 in]
      n104 = timed-loop "TestDriveLoop" {
        tunnel: w222 -> [w285]
        tunnel: w220 -> [w289]
        timing: w225 -> [_]
        timing-out: [_] -> w224
        stop <- FALSE stop-if-true
        w242 = 0.0 ("Dead Zone")
        (unwired) TRUE ("Quick Turn")
        # "PID Test"
        n105 = node-c288() -> (→"Late?":bool)  [unwired: 1 in]
        n106 = call <vilib>:"WPI_JoystickGetValues.vi"("JoystickDevRef"=w289) -> ("Buttons"=w263:bool[], "Axes"=w288:dbl[])  [unwired: 6 in, 3 out]
        n107 = Array To Cluster(array=w263) -> (cluster=w279:T35)
        n108 = Unbundle By Name(w279) -> ("Buttons[0]"=w227:bool, "Buttons[1]"=w246:bool, "Buttons[2]"=w244:bool)
        n109 = Select(t=DriveTypes."Auto Straight", s=w244, f=DriveTypes."Auto Turn") -> (s? t:f=w247:T11)
        n110 = Select(t=DriveTypes."Auto Vision Align", s=w246, f=w247) -> (s? t:f=w250:T11)
        "Drive Mode 2" <- w250
        n111 = Array To Cluster(array=w288) -> (cluster=w287:T36)
        n112 = Unbundle By Name(w287) -> ("Axes[1]"=w241:dbl, "Axes[2]"=w239:dbl)
        n113 = shared-variable ".\\Shared.lvlib\\IMU Yaw"() -> (w251:dbl)  [unwired: 1 in, 1 out]
        n114 = local read "Dead Zone"() -> (w236:dbl)
        n115 = call <userlib>:"Deadzone.vi"("Deadzone"=w236, "Input Signal"=w241) -> ("Output Signal"=w240:dbl)  [unwired: 1 out]
        n116 = Sign(1:w240) -> (0:w281:dbl)
        n117 = Square(x=w240) -> (x^2=w280:dbl)
        n118 = Multiply(x=w280, y=w281) -> (x*y=w268:dbl)
        n119 = Compound Arithmetic op=OR(w227, w244, w246) -> (w226:bool)
        n120 = case shown="\"Auto Straight\"" w250 {
          tunnel: [w305 w331 w342] -> w258
          tunnel: w251 -> [w311 w330 w350]
          tunnel: [0.0 ("Distance Setpoint") w329 0.0 ("Distance Setpoint")] -> w276
          tunnel: [0.0 ("Current Distance") w320 0.0 ("Current Distance")] -> w275
          tunnel: "PID Constants" -> [w313 w317 w346]
          tunnel: "Negates" -> [w309 w326 w352]
          tunnel: [w307 w325 w341] -> w267
          tunnel: [0.0 ("Cheesy Throttle") w318 0.0 ("Cheesy Throttle")] -> w266
          tunnel: "Angle Wrap" -> [_ w322 _]
          tunnel: w226 -> [w302 w321 _]
          frame "Auto Turn", Default {
            n121 = Unbundle By Name(w309) -> ("negate turn"=w308:bool)
            n122 = Unbundle By Name(w313) -> ("TurnPID"=w312:T37)
            n123 = call "Turn.vi"("Delta?"=TRUE, "Start Turn"=w302, "output range"="output range", "Negate"=w308, "PID gains"=w312, "Desired Angle"="Angle Delta", "Current Angle"=w311) -> ("Delta Angle Remaining"=→"Delta Angle Remaining":dbl, "Setpoint"=w305:dbl, "Cheesy Steer"=w307:dbl)  [unwired: 1 in, 1 out]
          }
          frame "Auto Straight" {
            n124 = shared-variable ".\\Shared.lvlib\\Encoder Distance"() -> (w320:dbl)  [unwired: 1 in, 1 out]
            n125 = Unbundle By Name(w317) -> ("Drive Distance PID"=w316:T37, "Drive Straight PID"=w315:T37)
            n126 = Bundle By Name(cluster=T34 {"Delta"=0.0, "Throttle Scale"=0.0, "Current Angle"=0.0, "Current Distance"=0.0} ("Drive Values"), "Delta"="Distance Delta", "Throttle Scale"="Throttle Scale", "Current Angle"=w330, "Current Distance"=w320) -> (w323:T34)
            n127 = Bundle("Drive Distance PID"=w316, "Drive Straight PID"=w315) -> (w314:T38)  [unwired: 1 in]
            n128 = call "DriveStraightExact.vi"("Angle Wrap"=w322, "Start Drive Straight (Hold)"=w321, "Negates"=w326, "PID Constants"=w314, "Drive Values"=w323) -> ("Setpoints"=w327:T39, "Cheesy Steer"=w325:dbl, "Cheesy Throttle"=w319:dbl)  [unwired: 4 in]
            n129 = Unbundle By Name(w327) -> ("Angle Setpoint"=w331:dbl, "Distance Setpoint"=w329:dbl)
            n130 = Negate(x=w319) -> (-x=w318:dbl)
          }
          frame "Auto Vision Align" {
            n131 = Unbundle By Name(w352) -> ("negate turn"=w351:bool)
            n132 = shared-variable ".\\Vision Variables.lvlib\\Right Target"() -> (w337:dbl)  [unwired: 1 in, 1 out]
            n133 = shared-variable ".\\Vision Variables.lvlib\\Left Target"() -> (w338:dbl)  [unwired: 1 in, 1 out]
            n134 = Unbundle By Name(w346) -> ("TurnPID"=w345:T37)
            n135 = shared-variable ".\\Vision Variables.lvlib\\Valid"() -> (w348:bool)  [unwired: 1 in, 1 out]
            n136 = Select(t=w338, s=TRUE, f=w337) -> (s? t:f=w336:dbl)
            n137 = Select(t=w336, s=w348, f=0.0) -> (s? t:f=w349:dbl)
            n138 = call "Turn.vi"("Delta?"=FALSE, "Start Turn"=FALSE, "Negate"=w351, "PID gains"=w345, "Desired Angle"=w349, "Current Angle"=w350) -> ("Delta Angle Remaining"=→"Delta Angle Remaining 3":dbl, "Setpoint"=w342:dbl, "Cheesy Steer"=w341:dbl)  [unwired: 2 in, 1 out]
          }
        }
        n139 = call <userlib>:"Deadzone.vi"("Deadzone"="Dead Zone 2", "Input Signal"=w239) -> ("Output Signal"=w238:dbl)  [unwired: 1 out]
        n140 = Sign(1:w238) -> (0:w283:dbl)
        n141 = Square(x=w238) -> (x^2=w284:dbl)
        n142 = Multiply(x=w284, y=w283) -> (x*y=w282:dbl)
        n143 = Negate(x=w282) -> (-x=w269:dbl)
        n144 = Array To Cluster(array=w263) -> (cluster=w264:T35)
        n145 = Unbundle By Name(w264) -> ("Buttons[7]"=w262:bool)
        n146 = Select(t=w267, s=w226, f=w269) -> (s? t:f=w228:dbl)
        n147 = Select(t=w266, s=w226, f=w268) -> (s? t:f=w265:dbl)
        n148 = case shown="True" w262 {
          tunnel: [w297 w298] -> w229
          tunnel: w265 -> [w296 w298]
          frame False {
            n149 = call-poly <vilib>:"PID Output Rate Limiter.vi"("output rate (EGU/min)"="output rate (EGU/min)", "input (controller output)"=w296) -> ("output"=w297:dbl)  [unwired: 6 in, 1 out]
          }
          frame True {
          }
        }
        n150 = Bundle("Distance Setpoint"=w276, "Current Distance"=w275) -> (→"Distance":T40)  [unwired: 1 in]
        n151 = Bundle("Setpoint"=w258, "Double"=w251) -> (→"Angle":cluster{"Setpoint":dbl, "Double":dbl})  [unwired: 1 in]
        n152 = local read "Offset"() -> (w243:dbl)
        n153 = call "Motor Adjustment.vi"("Offset"=w243, "Dead Zone"=w242, "X in"=w229) -> ("X Out"=w230:dbl)  [unwired: 8 in]
        n154 = call "Motor Adjustment.vi"("Offset"="Offset 2", "Dead Zone"=w242, "X in"=w228) -> ("X Out"=w231:dbl)  [unwired: 8 in]
        n155 = Subtract(x=w258, y=w251) -> (x-y=w257:dbl)
        n156 = Absolute Value(x=w257) -> (abs(x)=w256:dbl)
        n157 = Less Or Equal?(x=w256, y="tol") -> (x <= y?=w254:bool)
        n158 = Select(t=w228, s=w226, f=w231) -> (s? t:f=w232:dbl)
        n159 = Select(t=w229, s=w226, f=w230) -> (s? t:f=w233:dbl)
        n160 = call "Cheesy_drive.vi"("Quick Turn"=TRUE, "Wheel"=w232, "Throttle"=w233) -> ("Drive Data"=w272:cluster{"Left":dbl, "Right":dbl})  [unwired: 8 in]
        n161 = Unbundle By Name(w272) -> ("Left"=w271:dbl, "Right"=w270:dbl)
        n162 = call <userlib>:"De-Bounce or Delay.vi"("Eval Period (sec)"="Eval Period (sec)", "Signal Input"=w254) -> ("Stable"=→"Shoot":bool)  [unwired: 9 in]
        n163 = node-c288("Period") -> ()  [unwired: 1 out]
        n164 = call <vilib>:"WPI_RobotDriveTankDrive.vi"("Right axis value"=w270, "Left axis value"=w271, "RobotDriveDevRef"=w285) -> ()  [unwired: 6 in, 3 out]
      }
      n165 = node-c288(w224) -> ()  [unwired: 1 out]
    }
    frame Enabled {
    }
  }
  n166 = while {
    tunnel: "AutoQCP.csv" ("File Path") -> [w360]
    i -> [w359]
    stop <- FALSE stop-if-true
    n167 = Wait (ms)(milliseconds to wait=u32 100) -> ()  [unwired: 1 out]
    n168 = Less Or Equal?(x=w359, y=10) -> (x <= y?=w357:bool)
    n169 = Or(x=w357, y="Reload QCP") -> (x .or. y?=w355:bool)
    n170 = case shown="True" w355 {
      tunnel: w360 -> [_ w364]
      frame False {
      }
      frame True {
        n171 = call "QCP Reader.vi"("Path Relative?"=TRUE, "File Path"=w364) -> ()  [unwired: 10 in]
      }
    }
  }
  n172 = node-c288(i64 20 ("Period")) -> (w70:T20)  [unwired: 3 in]
  n173 = timed-loop "Drive Loop, Competition" {
    timing: w70 -> [_]
    timing-out: [_] -> w69
    tunnel: w67 -> [w379]
    tunnel: w65 -> [w375]
    tunnel: w62 -> [w376]
    tunnel: w36 -> [w374]
    stop <- FALSE stop-if-true
    n174 = node-c288() -> ()  [unwired: 1 in, 1 out]
    n175 = disable-structure shown="Disabled" {
      frame Disabled {
        (unwired) WPI_DriverStationRobotMode2."Autonomous Disabled" ("Robot Mode")
      }
      frame Enabled {
      }
    }
    n176 = shared-variable ".\\Shared.lvlib\\Robot Mode"() -> (w370:u32)  [unwired: 1 in, 1 out]
    n177 = shared-variable ".\\Shared.lvlib\\Encoder Distance"() -> (w371:dbl)  [unwired: 1 in, 1 out]
    n178 = local read "PID Constants"() -> (w365:T12)
    n179 = shared-variable ".\\Shared.lvlib\\IMU Yaw"() -> (w373:dbl)  [unwired: 1 in, 1 out]
    n180 = Select(t=w370, s="real mode", f="Drive Mode") -> (s? t:f=w367:u32)
    n181 = case shown="1" w367 {
      tunnel: w379 -> [_ _ _]
      tunnel: [w411 w468 w483] -> w378
      tunnel: [w410 w468 w482] -> w377
      tunnel: w376 -> [w427 _ _]
      tunnel: w375 -> [_ _ w485]
      tunnel: w374 -> [_ _ w484]
      tunnel: w373 -> [w393 _ w477]
      tunnel: w371 -> [w388 _ w481]
      tunnel: w365 -> [w408 _ w469]
      frame 3 {
        n182 = call <vilib>:"WPI_JoystickGetValues.vi"("JoystickDevRef"=w427) -> ("Buttons"=w384:bool[], "Axes"=w417:dbl[], "POVs"=w404:i16[])  [unwired: 6 in, 2 out]
        n183 = Index Array(array=w417, index #1=1 ("index"), index #2=2 ("index")) -> (element #1=w424:dbl, element #2=w423:dbl)
        n184 = call "Motor Adjustment.vi"("Offset"="Offset", "Dead Zone"="Dead Zone", "X in"=w424) -> ("X Out"=w420:dbl)  [unwired: 8 in]
        n185 = call "Motor Adjustment.vi"("Offset"="Offset", "Dead Zone"="Dead Zone", "X in"=w423) -> ("X Out"=w407:dbl)  [unwired: 8 in]
        n186 = Multiply(x="Max Val", y=w407) -> (x*y=w418:dbl)
        n187 = Multiply(x="Max Val", y=w420) -> (x*y=w413:dbl)
        n188 = Index Array(array=w404, index=0) -> (element=w402:i16)
        n189 = Not Equal To 0?(x=w413) -> (x != 0?=w399:bool)
        n190 = Not Equal To 0?(x=w407) -> (x != 0?=w396:bool)
        n191 = Equal?(x=w402, y=i16 0) -> (x = y?=w397:bool)
        n192 = Equal?(x=w402, y=i16 180) -> (x = y?=w395:bool)
        n193 = Not(x=w395) -> (.not. x?=w406:bool)
        n194 = Or(x=w396, y=w395) -> (x .or. y?=w394:bool)
        n195 = Compound Arithmetic op=OR(w399, w396, w397) -> (w398:bool)
        n196 = Index Array(array=w384, index=9) -> (element=w382:bool)
        n197 = call "JK Latch.vi"("Reset"=w394, "Set"=w397) -> ("Q"=w391:bool)  [unwired: 5 in]
        n198 = And(x=w398, y=w406) -> (x .and. y?=w405:bool)
        n199 = call "JK Latch.vi"("Reset"=w405, "Set"=w395) -> ("Q"=w392:bool)  [unwired: 5 in]
        n200 = Negate(x=w418) -> (-x=w414:dbl)
        n201 = Or(x=w392, y=w391) -> (x .or. y?=w389:bool)
        n202 = call "Sample And Hold.vi"("Signal"=w388, "Condition"=w389) -> ("Signal Out"=w387:dbl)  [unwired: 9 in]
        n203 = call "Sample And Hold.vi"("Signal"=w393, "Condition"=w389) -> ("Signal Out"=w390:dbl)  [unwired: 9 in]
        n204 = case shown="True" w392 {
          selector: w392 -> [_ w457]
          tunnel: [w449 w464] -> w416
          tunnel: w413 -> [w449 _]
          tunnel: [w448 w461] -> w415
          tunnel: w414 -> [w448 _]
          tunnel: w408 -> [_ w466]
          tunnel: w393 -> [_ w462]
          tunnel: w388 -> [_ w451]
          tunnel: w393 -> [_ w459]
          tunnel: w390 -> [_ w456]
          tunnel: w387 -> [_ w452]
          frame False {
          }
          frame True {
            n205 = Unbundle By Name(w466) -> ("Hold Position PID"=w465:T37, "TurnPID"=w460:T37)
            n206 = Subtract(x=w451, y=w452) -> (x-y=w450:dbl)
            n207 = Bundle By Name(cluster=T34 {"Delta"=0.0, "Throttle Scale"=1.0, "Current Angle"=0.0, "Current Distance"=0.0} ("Drive Values"), "Current Angle"=w462, "Current Distance"=w450) -> (w463:T34)
            n208 = call "Turn.vi"("Delta?"=FALSE, "Start Turn"=w457, "Negate"=TRUE, "PID gains"=w460, "Desired Angle"=w456, "Current Angle"=w459) -> ("Cheesy Steer"=w461:dbl)  [unwired: 2 in, 3 out]
            n209 = call "DriveDistance.vi"("Start Drive Straight (Hold)"=w457, "Negate"=TRUE, "Drive PID"=w465, "Drive Values"=w463) -> ("Distance Remaining"=→"Distance Remaining 2":dbl, "Cheesy Throttle"=w464:dbl)  [unwired: 6 in]
          }
        }
        n210 = case shown="True" w391 {
          tunnel: [w438 w446] -> w381
          tunnel: w416 -> [w438 w446]
          tunnel: w415 -> [w437 _]
          tunnel: [w437 w447] -> w385
          tunnel: w393 -> [_ w443]
          tunnel: w408 -> [_ w441]
          tunnel: w390 -> [_ w440]
          frame False {
          }
          frame True {
            n211 = Unbundle By Name(w441) -> ("Drive Straight PID"=w442:T37)
            n212 = call "Turn.vi"("Delta?"=FALSE, "Start Turn"=TRUE, "Negate"=TRUE, "PID gains"=w442, "Desired Angle"=w440, "Current Angle"=w443) -> ("Cheesy Steer"=w447:dbl)  [unwired: 2 in, 3 out]
          }
        }
        n213 = case shown="True" w382 {
          tunnel: [w429 w436] -> w386
          tunnel: w385 -> [w429 w436]
          tunnel: w381 -> [w428 _]
          tunnel: [w428 w435] -> w380
          frame False {
          }
          frame True {
            n214 = shared-variable ".\\Shared.lvlib\\Sonar"() -> (w434:dbl)  [unwired: 1 in, 1 out]
            n215 = Greater?(x=w434, y="dist away") -> (0:w432:bool)
            n216 = Select(t="a parameter too", s=w432, f=0.0) -> (s? t:f=w435:dbl)
          }
        }
        n217 = call <userlib>:"hmi_cheesy_drive.vi"("Quick Turn"=TRUE, "Wheel"=w386, "Throttle"=w380) -> ("Drive Data"=w412:cluster{"Left":dbl, "Right":dbl})  [unwired: 8 in]
        n218 = Unbundle By Name(w412) -> ("Left"=w411:dbl, "Right"=w410:dbl)
      }
      frame 0, Default {
        w468 = 0.0 ("Left Drive Motor")
      }
      frame 1 {
        n219 = shared-variable ".\\Vision Variables.lvlib\\Camera Delta"() -> (w478:dbl)  [unwired: 1 in, 1 out]
        n220 = Bundle("Double"=w478, "Double"=w477) -> (w476:cluster{"Double":dbl, "Double":dbl})  [unwired: 1 in]
        n221 = call "PeriodicTasksforSimulation.vi"("Distance (Based on Encoder)"=w481, "Gyro"=w477, "PID Constants"=w469, "notifier out 2"=w484, "notifier out"=w485, "Tollerances"="Tollerances") -> ("Right Drive Motor"=w482:dbl, "Left Drive Motor"=w483:dbl, "Command"=w471:T7, "Delta Angle Remaining"=→"Delta Angle Remaining 2":dbl, "Distance Remaining"=w470:dbl)  [unwired: 1 in]
        "Auto Command" <- w471
        "Distance Remaining" <- w470
        n222 = shared-variable ".\\Shared.lvlib\\Distance Remaining"(w470) -> ()  [unwired: 1 in, 1 out]
        n223 = Equal?(x=DriveStates."Follow Camera", y=w471) -> (x = y?=w472:bool)
        n224 = shared-variable ".\\Shared.lvlib\\AutoPeriodicCommands"(w471) -> ()  [unwired: 1 in, 1 out]
        n225 = Select(t=w476, s=w472, f=cluster{"Double":dbl, "Double":dbl} {"Double"=0.0, "Double"=0.0}) -> (s? t:f=→"Waveform Chart":cluster{"Double":dbl, "Double":dbl})
      }
    }
    n226 = call <vilib>:"WPI_RobotDriveTankDrive.vi"("Right axis value"=w377, "Left axis value"=w378, "RobotDriveDevRef"=w379) -> ()  [unwired: 6 in, 3 out]
    n227 = call "Elapsed Times.vi"("Call Name"="Drive") -> ()  [unwired: 2 in, 1 out]
    n228 = node-c288() -> ()  [unwired: 1 in, 1 out]
  }
  n229 = node-c288(w93) -> ()  [unwired: 1 out]
  n230 = call "IMUOrientRefNum Registry Get.vi"("refnum name"="Pri IMU") -> ("I2CDevRef out"=w60:T41)  [unwired: 9 in, 1 out]
  n231 = call <vilib>:"WPI_GyroRefNum Registry Get.vi"("refnum name"="Gyro") -> ("GyroDevRef"=w98:T43)  [unwired: 9 in, 1 out]
  n232 = call <vilib>:"WPI_GyroRefNum Registry Get.vi"("refnum name"="Pitch Gyro") -> ("GyroDevRef"=w40:T43)  [unwired: 9 in, 1 out]
  n233 = call "IMUOrientRefNum Registry Get.vi"("refnum name"="Alt IMU") -> ("I2CDevRef out"=w6:T41)  [unwired: 9 in, 1 out]
  n234 = Obtain Notifier(name (unnamed)="Climb Control", notification data type=Pneumatic_Commands."Nothing") -> (notifier out=w17:refnum<notifier>)  [unwired: 2 in, 2 out]
  n235 = call <vilib>:"WPI_MotorControlRefNum Registry Get.vi"("refnum name"="Winch") -> ("error out"=w31:errorcluster, "MotorControlDevRef"=w32:T27)  [unwired: 9 in]
  n236 = call <vilib>:"WPI_JoystickRefNum Registry Get.vi"("refnum name"="operatorJoystick") -> ("error out"=w33:errorcluster, "JoystickDevRef"=w34:T24)  [unwired: 9 in]
  n237 = call <vilib>:"WPI_ServoRefNum Registry Get.vi"("refnum name"="Climb Release") -> ("error out"=w14:errorcluster, "ServoDeviceRef"=w15:T46)  [unwired: 9 in]
  n238 = while {
    tunnel: w34 -> [w524]
    tunnel: w33 -> [w523]
    tunnel: w32 -> [w514]
    tunnel: w31 -> [w513]
    tunnel: w15 -> [w505]
    tunnel: w14 -> [w506]
    tunnel: w17 -> [w495]
    stop <- FALSE stop-if-true
    n239 = call <vilib>:"WPI_JoystickGetValues.vi"("error in (no error)"=w523, "JoystickDevRef"=w524) -> ("Buttons"=w522:bool[], "POVs"=w510:i16[])  [unwired: 5 in, 3 out]
    n240 = Index Array(array=w510) -> (element=w508:i16)  [unwired: 1 in]
    n241 = local read "Climb State"() -> (w493:T2)
    n242 = Index Array(array=w522, index #1=4 ("index"), index #2=5 ("index"), index #3=2 ("index"), index #4=1 ("index"), index #5=3 ("index")) -> (element #1=w500:bool, element #2=w499:bool, element #3=w517:bool, element #4=w494:bool, element #5=w496:bool)
    n243 = Or(x=w494, y=w496) -> (x .or. y?=w491:bool)
    n244 = Equal?(x=w493, y=Pneumatic_State_Machine."Up and Float") -> (x = y?=w490:bool)
    n245 = And(x=w500, y=w499) -> (x .and. y?=w489:bool)
    n246 = Equal To 0?(x=w508) -> (x = 0?=w509:bool)
    n247 = Select(t=1.0 ("Winch"), s=w517, f=0.0) -> (s? t:f=w512:dbl)
    n248 = case shown="True" w491 {
      tunnel: w495 -> [_ w529]
      tunnel: w494 -> [_ w525]
      frame False {
      }
      frame True {
        n249 = Select(t=Pneumatic_Commands."Go Up", s=w525, f=Pneumatic_Commands."Go Down") -> (s? t:f=w526:T17)
        n250 = Send Notification(notification=w526, notifier=w529) -> ()  [unwired: 1 in, 2 out]
      }
    }
    n251 = And(x=w489, y=w490) -> (x .and. y?=w488:bool)
    n252 = Select(t=-1.0, s=w509, f=w512) -> (s? t:f=w511:dbl)
    n253 = call <userlib>:"Latch.vi"("In"=w488) -> ("Out"=w504:bool)  [unwired: 1 in]
    n254 = call <vilib>:"WPI_MotorControlSetOutput.vi"("error in (no error)"=w513, "Output"=w511, "MotorControlDevRef"=w514) -> ()  [unwired: 6 in, 3 out]
    n255 = Select(t=50, s=w504, f=10) -> (s? t:f=w502:i32)
    n256 = call <vilib>:"WPI_ServoSetAngle.vi"("error in (no error)"=w506, "Angle"=w502, "ServoDeviceRef"=w505) -> ()  [unwired: 7 in, 2 out]
  }
  n257 = call <vilib>:"WPI_SolenoidRefNum Registry Get.vi"("refnum name"="Climb") -> ("error out"=w27:errorcluster, "SolenoidDevRef"=w25:T47)  [unwired: 9 in]
  n258 = call-poly <vilib>:"WPI_SolenoidSet.vi"("error in (no error)"=w27, "Value"=WPI_SolenoidValue."Forward", "SolenoidDevRef"=w25) -> ("error out"=w28:errorcluster, "SolenoidDevRef"=w26:T47)  [unwired: 7 in]
  n259 = Obtain Notifier(name (unnamed)="Climb Control", notification data type=Pneumatic_Commands."Nothing") -> (notifier out=w23:refnum<notifier>)  [unwired: 2 in, 2 out]
  n260 = node-c288() -> (w102:T20)  [unwired: 4 in]
  n261 = timed-loop "IMU Loop, Time Critical" {
    timing: w102 -> [_]
    timing-out: [_] -> w101
    tunnel: w60 -> [w548]
    tunnel: w98 -> [w545]
    tunnel: w40 -> [w543]
    shift-right: [w538] -> _
    shift-left: IMUType."Pri IMU" -> [w540]
    shift-right: [w537] -> _
    shift-left: T15 {"Yaw Wind"=0.0, "Roll Wind"=0.0, "Pitch Wind"=0.0} -> [w536]
    tunnel: w6 -> [w535]
    stop <- _ stop-if-true
    n262 = node-c288() -> (→"Late? 2":bool)  [unwired: 1 in]
    n263 = Unbundle By Name(w548) -> ("DevStatus.status"=→"IMUStatus":bool)
    n264 = call <vilib>:"WPI_GyroGetAngle.vi"("GyroDevRef"=w543) -> ("Angle"=w541:dbl)  [unwired: 6 in, 4 out]
    n265 = Negate(x=w541) -> (-x=w530:dbl)
    "Analog Pitch Gyro 2" <- w530
    n266 = call <vilib>:"WPI_GyroGetAngle.vi"("GyroDevRef"=w545) -> ("Angle"=w544:dbl)  [unwired: 6 in, 4 out]
    n267 = case shown="\"Pri IMU\", Default" w540 {
      selector: w540 -> [w567 w617 _]
      tunnel: w548 -> [w595 _ _]
      tunnel: [w584 w634 w651] -> w547
      tunnel: w544 -> [w554 w603 w656]
      tunnel: [w552 w601 w650] -> w542
      tunnel: w530 -> [_ _ w655]
      tunnel: [w568 w618 IMUType."Analog GYRO"] -> w538
      tunnel: [w560 w610 _] -> w537
      tunnel: w536 -> [w559 w609 w654]
      tunnel: w535 -> [_ w604 _]
      tunnel: [w554 w603 w651] -> w534
      tunnel: [w553 w602 w651] -> w533
      tunnel: [w552 w601 w650] -> w532
      tunnel: [w551 w600 0.0 ("Pitch Wind")] -> w531
      frame "Pri IMU", Default {
        n268 = First Call?() -> (First Call?: T/F=w558:bool)
        n269 = call "IMUOrientRead.vi"("I2CDevRef"=w595, "Orient Reset"=w558, "Read Enable"="Read Enable", "Orient Ref"=w559, "Earth Field (uT)"="Earth Field (uT)") -> ("Cal Status"=w598:T49, "Orient Y/R/P"=w561:T50, "Acc X,Y,Z"=w597:cluster{"X Acc":dbl, "Y Acc":dbl, "Z Acc":dbl}, "Mag Field X,Y,Z"=w585:T51)  [unwired: 4 in, 3 out]
        n270 = Unbundle By Name(w585) -> ("X Mag"=w587:dbl, "Y Mag"=w588:dbl, "Z Mag"=w589:dbl, "Anomaly"=→"Anomaly":bool)
        n271 = Unbundle(w598) -> ("Mag"=w580:T52, "Acc"=w575:T52, "Gyro"=w574:T52, "Sys"=w573:T52, "Status"=w566:bool)
        "S" <- w573
        "G" <- w574
        "A" <- w575
        "M" <- w580
        n272 = Unbundle By Name(w561) -> ("Yaw Wind"=w584:dbl, "Yaw Wind"=w553:dbl, "Roll Wind"=w552:dbl, "Pitch Wind"=w551:dbl)
        "pitch" <- w552
        n273 = Unbundle By Name(w597) -> ("X Acc"=w583:dbl, "Y Acc"=w582:dbl, "Z Acc"=w581:dbl)
        "X Acc" <- w583
        "Y Acc" <- w582
        "Z Acc" <- w581
        n274 = Cluster To Array(cluster=w580) -> (array=w579:bool[])
        n275 = Boolean Array To Number(Boolean array=w579) -> (number=w571:u32)
        n276 = Square(x=w589) -> (x^2=w590:dbl)
        n277 = Square(x=w587) -> (x^2=w591:dbl)
        n278 = Square(x=w588) -> (x^2=w592:dbl)
        n279 = Compound Arithmetic op=ADD(w590, w591, w592) -> (w593:dbl)
        n280 = Cluster To Array(cluster=w575) -> (array=w578:bool[])
        n281 = Square Root(x=w593) -> (sqrt(x)=→"Mag Vector":dbl)
        n282 = Boolean Array To Number(Boolean array=w578) -> (number=w570:u32)
        n283 = Cluster To Array(cluster=w574) -> (array=w577:bool[])
        n284 = Boolean Array To Number(Boolean array=w577) -> (number=w569:u32)
        n285 = shared-variable ".\\Shared.lvlib\\IMU Roll"(w551) -> ()  [unwired: 1 in, 1 out]
        n286 = Cluster To Array(cluster=w573) -> (array=w576:bool[])
        n287 = shared-variable ".\\Shared.lvlib\\Accel X"(w583) -> ()  [unwired: 1 in, 1 out]
        n288 = shared-variable ".\\Shared.lvlib\\Accel Y"(w582) -> ()  [unwired: 1 in, 1 out]
        n289 = shared-variable ".\\Shared.lvlib\\Accel Z"(w581) -> ()  [unwired: 1 in, 1 out]
        n290 = shared-variable ".\\Shared.lvlib\\IMU Cal M"(w571) -> ()  [unwired: 1 in, 1 out]
        n291 = Boolean Array To Number(Boolean array=w576) -> (number=w572:u32)
        n292 = shared-variable ".\\Shared.lvlib\\IMU Cal G"(w569) -> ()  [unwired: 1 in, 1 out]
        n293 = shared-variable ".\\Shared.lvlib\\IMU Cal A"(w570) -> ()  [unwired: 1 in, 1 out]
        n294 = Not(x=w566) -> (.not. x?=w555:bool)
        n295 = shared-variable ".\\Shared.lvlib\\IMU Cal S"(w572) -> ()  [unwired: 1 in, 1 out]
        n296 = Unbundle By Name(w561) -> ("Yaw Wind"=w564:dbl, "Roll Wind"=w563:dbl, "Pitch Wind"=w562:dbl)
        n297 = Or(x="PImu fail", y=w555) -> (x .or. y?=w557:bool)
        n298 = Bundle("Yaw Wind"=w564, "Roll Wind"=w563, "Pitch Wind"=w562) -> (w560:T15)  [unwired: 1 in]
        n299 = Select(t=IMUType."Alt IMU", s=w557, f=w567) -> (s? t:f=w568:T1)
      }
      frame "Alt IMU" {
        n300 = First Call?() -> (First Call?: T/F=w608:bool)
        n301 = call "IMUOrientRead.vi"("I2CDevRef"=w604, "Orient Reset"=w608, "Read Enable"="Read Enable 2", "Orient Ref"=w609, "Earth Field (uT)"="Earth Field (uT) 2") -> ("Cal Status"=w647:T49, "Orient Y/R/P"=w611:T50, "Acc X,Y,Z"=w646:cluster{"X Acc":dbl, "Y Acc":dbl, "Z Acc":dbl}, "Mag Field X,Y,Z"=w635:T51)  [unwired: 4 in, 3 out]
        n302 = Unbundle By Name(w635) -> ("X Mag"=w637:dbl, "Y Mag"=w638:dbl, "Z Mag"=w639:dbl, "Anomaly"=→"Anomaly 2":bool)
        n303 = Unbundle(w647) -> ("Mag"=w630:T52, "Acc"=w625:T52, "Gyro"=w624:T52, "Sys"=w623:T52, "Status"=w616:bool)
        "S 2" <- w623
        "G 2" <- w624
        "A 2" <- w625
        "M 2" <- w630
        n304 = Unbundle By Name(w611) -> ("Yaw Wind"=w634:dbl, "Yaw Wind"=w602:dbl, "Roll Wind"=w601:dbl, "Pitch Wind"=w600:dbl)
        "pitch 2" <- w601
        n305 = Unbundle By Name(w646) -> ("X Acc"=w633:dbl, "Y Acc"=w632:dbl, "Z Acc"=w631:dbl)
        "X Acc 2" <- w633
        "Y Acc 2" <- w632
        "Z Acc 2" <- w631
        n306 = Cluster To Array(cluster=w630) -> (array=w629:bool[])
        n307 = Boolean Array To Number(Boolean array=w629) -> (number=w621:u32)
        n308 = Square(x=w639) -> (x^2=w640:dbl)
        n309 = Square(x=w637) -> (x^2=w641:dbl)
        n310 = Square(x=w638) -> (x^2=w642:dbl)
        n311 = Compound Arithmetic op=ADD(w640, w641, w642) -> (w643:dbl)
        n312 = Cluster To Array(cluster=w625) -> (array=w628:bool[])
        n313 = Square Root(x=w643) -> (sqrt(x)=→"Mag Vector 2":dbl)
        n314 = Boolean Array To Number(Boolean array=w628) -> (number=w620:u32)
        n315 = Cluster To Array(cluster=w624) -> (array=w627:bool[])
        n316 = Boolean Array To Number(Boolean array=w627) -> (number=w619:u32)
        n317 = shared-variable ".\\Shared.lvlib\\IMU Roll"(w600) -> ()  [unwired: 1 in, 1 out]
        n318 = Cluster To Array(cluster=w623) -> (array=w626:bool[])
        n319 = shared-variable ".\\Shared.lvlib\\Accel X"(w633) -> ()  [unwired: 1 in, 1 out]
        n320 = shared-variable ".\\Shared.lvlib\\Accel Y"(w632) -> ()  [unwired: 1 in, 1 out]
        n321 = shared-variable ".\\Shared.lvlib\\Accel Z"(w631) -> ()  [unwired: 1 in, 1 out]
        n322 = shared-variable ".\\Shared.lvlib\\IMU Cal M"(w621) -> ()  [unwired: 1 in, 1 out]
        n323 = Boolean Array To Number(Boolean array=w626) -> (number=w622:u32)
        n324 = shared-variable ".\\Shared.lvlib\\IMU Cal G"(w619) -> ()  [unwired: 1 in, 1 out]
        n325 = shared-variable ".\\Shared.lvlib\\IMU Cal A"(w620) -> ()  [unwired: 1 in, 1 out]
        n326 = shared-variable ".\\Shared.lvlib\\IMU Cal S"(w622) -> ()  [unwired: 1 in, 1 out]
        n327 = Not(x=w616) -> (.not. x?=w605:bool)
        n328 = Unbundle By Name(w611) -> ("Yaw Wind"=w614:dbl, "Roll Wind"=w613:dbl, "Pitch Wind"=w612:dbl)
        n329 = Or(x=w605, y="Alt imu") -> (x .or. y?=w607:bool)
        n330 = Bundle("Yaw Wind"=w614, "Roll Wind"=w613, "Pitch Wind"=w612) -> (w610:T15)  [unwired: 1 in]
        n331 = Select(t=IMUType."Analog GYRO", s=w607, f=w617) -> (s? t:f=w618:T1)
      }
      frame "Analog GYRO" {
        n332 = Unbundle By Name(w654) -> ("Yaw Wind"=w653:dbl, "Roll Wind"=w652:dbl)  [unwired: 1 out]
        n333 = Subtract(x=w655, y=w652) -> (x-y=w659:dbl)
        n334 = First Call?() -> (First Call?: T/F=w660:bool)
        n335 = feedback #2() -> (w658:dbl)  [unwired: 1 in]
        n336 = Select(t=w659, s=w660, f=w658) -> (s? t:f=w657:dbl)
        n337 = feedback-in #2(w657) -> ()
        n338 = Subtract(x=w655, y=w657) -> (x-y=w650:dbl)
        n339 = Subtract(x=w656, y=w653) -> (x-y=w662:dbl)
        n340 = First Call?() -> (First Call?: T/F=w661:bool)
        n341 = feedback #3() -> (w663:dbl)  [unwired: 1 in]
        n342 = Select(t=w662, s=w661, f=w663) -> (s? t:f=w664:dbl)
        n343 = feedback-in #3(w664) -> ()
        n344 = Subtract(x=w656, y=w664) -> (x-y=w651:dbl)
      }
    }
    "Analog Yaw Gyro" <- w534
    "Yaw" <- w533
    "Pitch" <- w532
    "Roll" <- w531
    "IMU Type" <- w538
    n345 = shared-variable ".\\Shared.lvlib\\IMU Pitch"(w542) -> ()  [unwired: 1 in, 1 out]
    n346 = shared-variable ".\\Shared.lvlib\\IMU Yaw"(w547) -> ()  [unwired: 1 in, 1 out]
    n347 = call "Elapsed Times.vi"("Call Name"="IMU") -> ()  [unwired: 2 in, 1 out]
    n348 = node-c288("Sensor Period") -> ()  [unwired: 1 out]
  }
  n349 = while "Intake Position Loop" {
    tunnel: w23 -> [w678]
    tunnel: w26 -> [w675]
    tunnel: w28 -> [w674]
    shift-right: [w673] -> _
    shift-left: Pneumatic_State_Machine."Down and Pressue" ("State Out") -> [w672]
    stop <- FALSE stop-if-true
    n350 = call "Pneumatic Controller.vi"("State In"=w672, "Time Limit Down"=0, "Time Limit Up"=0, "Notifier in"=w678) -> ("State Out"=w673:T2, "Value"=w671:T18)  [unwired: 6 in]
    "Climb State" <- w673
    n351 = call-poly <vilib>:"WPI_SolenoidSet.vi"("error in (no error)"=w674, "Value"=w671, "SolenoidDevRef"=w675) -> ()  [unwired: 7 in, 2 out]
  }
  n352 = call <vilib>:"WPI_SolenoidRefNum Registry Get.vi"("refnum name"="Intake Solenoid") -> ("error out"=w56:errorcluster, "SolenoidDevRef"=w58:T47)  [unwired: 9 in]
  n353 = call <vilib>:"WPI_SolenoidRefNum Registry Get.vi"("refnum name"="Tusks") -> ("error out"=w44:errorcluster, "SolenoidDevRef"=w46:T47)  [unwired: 9 in]
  n354 = call-poly <vilib>:"WPI_SolenoidSet.vi"("error in (no error)"=w56, "Value"=WPI_SolenoidValue."Reverse", "SolenoidDevRef"=w58) -> ("error out"=w55:errorcluster, "SolenoidDevRef"=w57:T47)  [unwired: 7 in]
  n355 = Obtain Notifier(name (unnamed)="Intake Control", notification data type=Pneumatic_Commands."Nothing") -> (notifier out=w87:refnum<notifier>)  [unwired: 2 in, 2 out]
  n356 = call-poly <vilib>:"WPI_SolenoidSet.vi"("error in (no error)"=w44, "Value"=WPI_SolenoidValue."Forward", "SolenoidDevRef"=w46) -> ("error out"=w43:errorcluster, "SolenoidDevRef"=w45:T47)  [unwired: 7 in]
  n357 = Obtain Notifier(name (unnamed)="Tusk Control", notification data type=Pneumatic_Commands."Nothing") -> (notifier out=w50:refnum<notifier>)  [unwired: 2 in, 2 out]
  n358 = while "Intake Position Loop" {
    tunnel: w87 -> [w688]
    tunnel: w57 -> [w685]
    tunnel: w55 -> [w684]
    shift-right: [w683] -> _
    shift-left: Pneumatic_State_Machine."Up and Pressure" ("State Out") -> [w682]
    stop <- FALSE stop-if-true
    n359 = call "Pneumatic Controller.vi"("State In"=w682, "Time Limit Down"=2000, "Time Limit Up"=2000, "Notifier in"=w688) -> ("State Out"=w683:T2, "Value"=w681:T18)  [unwired: 6 in]
    "Intake State" <- w683
    n360 = call-poly <vilib>:"WPI_SolenoidSet.vi"("error in (no error)"=w684, "Value"=w681, "SolenoidDevRef"=w685) -> ()  [unwired: 7 in, 2 out]
    n361 = To Double Precision Float(number=w681) -> (double precision float=→"Intake Chart":dbl)
  }
  n362 = while "Intake Position Loop" {
    tunnel: w50 -> [w697]
    tunnel: w45 -> [w694]
    tunnel: w43 -> [w693]
    shift-right: [w692] -> _
    shift-left: Pneumatic_State_Machine."Down and Pressue" ("State Out") -> [w691]
    stop <- FALSE stop-if-true
    n363 = call "Pneumatic Controller.vi"("State In"=w691, "Time Limit Down"=2000, "Time Limit Up"=2000, "Notifier in"=w697) -> ("State Out"=w692:T2, "Value"=w690:T18)  [unwired: 6 in]
    "Tusk State" <- w692
    n364 = call-poly <vilib>:"WPI_SolenoidSet.vi"("error in (no error)"=w693, "Value"=w690, "SolenoidDevRef"=w694) -> ()  [unwired: 7 in, 2 out]
  }
  n365 = Type Cast(type=u32 0 ("milliseconds to wait"), x=w87) -> (*(type *) &x=w85:u32)
  n366 = Type Cast(type=u32 0 ("milliseconds to wait"), x=w50) -> (*(type *) &x=w48:u32)
  n367 = shared-variable ".\\Shared.lvlib\\Intake Notifier Typecast"(w85) -> ()  [unwired: 1 in, 1 out]
  n368 = shared-variable ".\\Shared.lvlib\\Tusks Notifier Typecast"(w48) -> ()  [unwired: 1 in, 1 out]
  n369 = node-c288(w69) -> ()  [unwired: 1 out]
  n370 = node-c288(w101) -> ()  [unwired: 1 out]
  n371 = call <vilib>:"WPI_EncoderRefNum Registry Get.vi"("refnum name"="Right Encoder") -> ("error out"=w79:errorcluster, "EncoderDevRef"=w80:T53)  [unwired: 9 in]
  n372 = call <vilib>:"WPI_EncoderRefNum Registry Get.vi"("refnum name"="Left Encoder") -> ("error out"=w78:errorcluster, "EncoderDevRef"=w77:T53)  [unwired: 9 in]
  n373 = node-c288(i64 20 ("Period")) -> (w84:T20)  [unwired: 3 in]
  n374 = while {
    stop <- FALSE stop-if-true
    n375 = local read "Analog Pitch Gyro 2"() -> (w699:dbl)
    n376 = local read "Analog Yaw Gyro"() -> (w701:dbl)
    n377 = local read "IMUStatus"() -> (w704:bool)
    n378 = shared-variable ".\\Shared.lvlib\\Right Encoder Distance"() -> (w709:dbl)  [unwired: 1 in, 1 out]
    n379 = Wait (ms)(milliseconds to wait=u32 100) -> ()  [unwired: 1 out]
    n380 = shared-variable ".\\Shared.lvlib\\Left Encoder Distance"() -> (w711:dbl)  [unwired: 1 in, 1 out]
    n381 = shared-variable ".\\Shared.lvlib\\IMU Yaw"() -> (w708:dbl)  [unwired: 1 in, 1 out]
    n382 = shared-variable ".\\Shared.lvlib\\Boulder Detected"() -> (w714:bool)  [unwired: 1 in, 1 out]
    n383 = shared-variable ".\\Shared.lvlib\\Sonar"() -> (w706:dbl)  [unwired: 1 in, 1 out]
    n384 = call-poly <vilib>:"NT Write Value.vi"("Numeric"=w708, "Name"="IMU Yaw") -> ()  [unwired: 9 in, 1 out]
    n385 = call-poly <vilib>:"NT Write Value.vi"("Numeric"=w701, "Name"="Analog Yaw Gyro") -> ()  [unwired: 9 in, 1 out]
    n386 = call-poly <vilib>:"NT Write Value.vi"("Numeric"=w699, "Name"="Analog Pitch Gyro") -> ()  [unwired: 9 in, 1 out]
    n387 = call-poly <vilib>:"NT Write Value.vi"("Boolean"=w704, "Name"="IMU Error") -> ()  [unwired: 9 in, 1 out]
    n388 = call-poly <vilib>:"NT Write Value.vi"("Numeric"=w706, "Name"="Sharp Sensor") -> ()  [unwired: 9 in, 1 out]
    n389 = call-poly <vilib>:"NT Write Value.vi"("Boolean"=w714, "Name"="Boulder Detected") -> ()  [unwired: 9 in, 1 out]
    n390 = call-poly <vilib>:"NT Write Value.vi"("Numeric"=w709, "Name"="Right Encoder") -> ()  [unwired: 9 in, 1 out]
    n391 = call-poly <vilib>:"NT Write Value.vi"("Numeric"=w711, "Name"="Left Encoder") -> ()  [unwired: 9 in, 1 out]
  }
  n392 = call <vilib>:"WPI_Power Get PDP Currents.vi"() -> ("all currents (A)"=w72:dbl[])  [unwired: 13 in, 2 out]
  n393 = Add Array Elements(numeric array=w72) -> (sum=w71:dbl)
  n394 = timed-loop "Encoder Loop" {
    timing: w84 -> [_]
    timing-out: [_] -> w83
    tunnel: w80 -> [w734]
    tunnel: w79 -> [w733]
    tunnel: w78 -> [w732]
    tunnel: w77 -> [w731]
    tunnel: w71 -> [w727]
    stop <- FALSE stop-if-true
    n395 = node-c288() -> ()  [unwired: 1 in, 1 out]
    n396 = call <vilib>:"WPI_Power Get PDP Currents.vi"() -> ("all currents (A)"=w723:dbl[])  [unwired: 13 in, 2 out]
    n397 = call "Elapsed Times.vi"("Call Name"="Encoder") -> ()  [unwired: 2 in, 1 out]
    n398 = Index Array(array=w723, index=6) -> (element=w721:dbl)
    n399 = call <vilib>:"WPI_EncoderGet.vi"("error in (no error)"=w732, "EncoderDevRef"=w731) -> ("Distance"=w717:dbl, "EncoderDevRef"=w726:T53)  [unwired: 4 in, 4 out]
    "Left Encoder Distance" <- w717
    n400 = Add Array Elements(numeric array=w723) -> (sum=w729:dbl)
    n401 = call <vilib>:"WPI_EncoderGet.vi"("error in (no error)"=w733, "EncoderDevRef"=w734) -> ("Distance"=w730:dbl, "EncoderDevRef"=w724:T53)  [unwired: 4 in, 4 out]
    "Right Encoder Distance" <- w730
    n402 = Subtract(x=w729, y=w727) -> (x-y=→"Motor Current":dbl)
    n403 = Greater?(x=w721, y=10.0) -> (0:w719:bool)
    n404 = case shown="True" "Reset Encoders" {
      tunnel: w726 -> [_ w737]
      tunnel: w724 -> [_ w736]
      frame False {
      }
      frame True {
        n405 = call <vilib>:"WPI_EncoderReset.vi"("EncoderDevRef"=w737) -> ()  [unwired: 9 in, 2 out]
        n406 = call <vilib>:"WPI_EncoderReset.vi"("EncoderDevRef"=w736) -> ()  [unwired: 9 in, 2 out]
      }
    }
    n407 = shared-variable ".\\Shared.lvlib\\Boulder Detected"(w719) -> ()  [unwired: 1 in, 1 out]
    n408 = shared-variable ".\\Shared.lvlib\\Right Encoder Distance"(w730) -> ()  [unwired: 1 in, 1 out]
    n409 = shared-variable ".\\Shared.lvlib\\Encoder Distance"(w717) -> ()  [unwired: 1 in, 1 out]
    n410 = shared-variable ".\\Shared.lvlib\\Left Encoder Distance"(w717) -> ()  [unwired: 1 in, 1 out]
    n411 = node-c288() -> ()  [unwired: 1 in, 1 out]
  }
  n412 = node-c288(w83) -> ()  [unwired: 1 out]
